vi "digital_demod_fpga.vi"() -> ()   [LabVIEW 2018]
uses:
  <vilib>/Platform/TimedLoop/XDataNode/timing_clust.ctl
  <vilib>/Platform/TimedLoop/XDataNode/nitl_modes.ctl
  <vilib>/Platform/TimedLoop/XDataNode/wakeup.ctl
  <vilib>/rvi/FXPMathLib/FxpAtan2/subVIs/nifxpmath_Atan2_SimConfig.ctl
  <vilib>/rvi/Emulation/niFpgaGetClockAttributes.vi
  <vilib>/rvi/Emulation/niFpgaSctlEmulationGetInTimedLoop.vi
  <vilib>/rvi/Emulation/niFpgaEmulationReportErrorSimple.vi
  <vilib>/rvi/Emulation/niFpgaCriticalErrorInLSC.vi
  <vilib>/rvi/Emulation/niFpgaProcessEmulError.vi
  <vilib>/rvi/eio/common/nirviEmuTemplateMethod_errors.vi
  <vilib>/rvi/DataTransferAndStorage/Container/Common/niFpgaContainerExecOnDevCompGetState.vi
  <vilib>/rvi/Emulation/niFpgaEmulationIsFPGAContextNoSignature.vi
  <vilib>/rvi/errors/niFpgaSetErrorForExecOnDevCompSimple.vi
  <vilib>/rvi/eio/common/nirviEmuReportErrorAndStop.vi
  <vilib>/rvi/DataTransferAndStorage/Container/Common/niFpgaContainerGetUniqueNameForEmu.vi
  <vilib>/rvi/FIFO/Fifo_Resource/nirvififoEmulationSetSize.vi
  <vilib>/rvi/FIFO/Fifo_Resource/nirviFifoEmulationQueueMgr.vi
  <instcachedir>/0/nirviFifoEmulationQueueMgr_E5CAEC123FF24DC58D834DCA3CDAA9B5.lvgen/nirviFifoEmulationQueueMgr_E5CAEC123FF24DC58D834DCA3CDAA9B5_006.vi
  <vilib>/rvi/FIFO/Fifo_Resource/nirvififoEmulationDetermineInputValidOut.vi
  <vilib>/rvi/FIFO/Fifo_Resource/nirvififoEmulationCreateLock.vi
  <vilib>/rvi/FIFO/Fifo_Resource/nirvififoEmulationObtainLock.vi
  <vilib>/rvi/FIFO/Fifo_Resource/nirvififoEmulationReleaseLock.vi
  <vilib>/rvi/occurrence/nirviWaitOnOccurrenceBase.vi
  <vilib>/rvi/errors/nirviReportUnexpectedCaseInternalError.vi
  <vilib>/rvi/errors/nirviReportUnexpectedCaseInternalError (U32).vi
  <vilib>/Utility/error.llb/Clear Errors.vi
  <vilib>/rvi/interface/RandomDataEmulation/niFpgaRandomDataHandleErrors.vi
  <instcachedir>/0/nirviFifoEmulationQueueMgr_E5CAEC123FF24DC58D834DCA3CDAA9B5.lvgen/nirviFifoEmulationQueueMgr_E5CAEC123FF24DC58D834DCA3CDAA9B5_001.vi
  <vilib>/rvi/Memory/Memory_Emulation/niFpgaMemoryEmulationCacheClearOnFirstRun.vi
  <vilib>/rvi/Memory/Memory_Emulation/nirvimemoryEmulationManagerCache_MakeExclusive.vi
  <vilib>/rvi/Memory/Memory_Emulation/niFpgaMemoryEmulationValidateCache.vi
  <vilib>/rvi/Memory/Memory_Emulation/nirvimemoryEmulationManagerCache_InsertValue.vi
  <vilib>/rvi/Memory/Memory_Emulation/nirvimemoryEmulationManagerCache_ReleaseExclusive.vi
  <vilib>/rvi/Memory/Memory_Emulation/nirvimemoryEmulationManagerCache_GetValue.vi
  <vilib>/rvi/Memory/Memory_Emulation/nirvimemoryEmulationManagerCache_SetValue.vi
  <vilib>/rvi/Emulation/niFpgaSctlEmulationResourceMgr.vi
  <instcachedir>/0/nirviFifoEmulationQueueMgr_E5CAEC123FF24DC58D834DCA3CDAA9B5.lvgen/nirviFifoEmulationQueueMgr_E5CAEC123FF24DC58D834DCA3CDAA9B5_003.vi
  <instcachedir>/0/nirviFifoEmulationQueueMgr_E5CAEC123FF24DC58D834DCA3CDAA9B5.lvgen/nirviFifoEmulationQueueMgr_E5CAEC123FF24DC58D834DCA3CDAA9B5_002.vi
  <instcachedir>/0/nirviFifoEmulationQueueMgr_E5CAEC123FF24DC58D834DCA3CDAA9B5.lvgen/nirviFifoEmulationQueueMgr_E5CAEC123FF24DC58D834DCA3CDAA9B5_004.vi
  <vilib>/rvi/FXPMathLib/FxpAtan2/simVIs/DllFxpAtan2Temp_sub.vi
  <instcachedir>/0/nirviFifoEmulationQueueMgr_E5CAEC123FF24DC58D834DCA3CDAA9B5.lvgen/nirviFifoEmulationQueueMgr_E5CAEC123FF24DC58D834DCA3CDAA9B5_009.vi
  <instcachedir>/0/nirviFifoEmulationQueueMgr_E5CAEC123FF24DC58D834DCA3CDAA9B5.lvgen/nirviFifoEmulationQueueMgr_E5CAEC123FF24DC58D834DCA3CDAA9B5_007.vi
  <instcachedir>/0/nirviFifoEmulationQueueMgr_E5CAEC123FF24DC58D834DCA3CDAA9B5.lvgen/nirviFifoEmulationQueueMgr_E5CAEC123FF24DC58D834DCA3CDAA9B5_008.vi
  <vilib>/Platform/TimedLoop/XDataNode/XDataNode.xnode
  <vilib>/eio/EIONode/EIONode.xnode
  <vilib>/rvi/DataTransferAndStorage/Container/XNode/niFpgaContainer.xnode
  <vilib>/rvi/FIFO/Fifo_Resource/niFpgaFifoEmulationRefIn.vi
  <vilib>/rvi/Memory/Memory_Emulation/niFpgaMemoryEmulationRefIn.vi
  <vilib>/rvi/FXPMathLib/FxpInterpret/XNode/nifxpmath_Interpret.xnode
  <vilib>/rvi/FXPMathLib/FxpAtan2/XNode/nifxpmath_Atan2.xnode
  <vilib>/Platform/TimedLoop/XDataNode/XDNodeRunTimeDep.lvlib
  FPGA Timekeeper 1.1b0/FPGA Timekeeper.lvlib
  <instrlib>/_niInstr_jank/Basic Elements/v1/FPGA/niInstr Basic Elements v1 FPGA.lvlib
panel:
  in  "sum_z-pow_fb":bool
  in  "pow_dc_offset":i16
  out "pow_set_actual":fxp<+/-,33,33>
  in  "fb_on_pow_set":bool
  in  "pow_fb":bool
  in  "pow_lower_lim":i16
  in  "pow_upper_lim":i16
  in  "pow_pg":fxp<+/-,32,16>
  in  "pow_dg":fxp<+/-,32,16>
  out "amp4_lf":i32
  out "delta_pow_set":fxp<+/-,32,32>
  in  "delta_pow_set_llim":fxp<+/-,32,32>
  in  "delta_pow_set_ulim":fxp<+/-,32,32>
  out "pow_shifted":i32
  in  "pow_fb_bitshift":i16
  in  "reset_pow_accum":bool
  in  "pow_ig":fxp<+/-,32,16>
  in  "pow_set_user":fxp<+/-,32,32>
  in  "pow_bitshift":i16
  out "z_fb_tot_i16":i16
  in  "z_internal_inject_scale":i16
  in  "add_sin":bool
  in  "z_internal_inject_freq":fxp<+,32,0>=0.0002500000409781933
  in  "inject_sigs":bool
  in  "downsample->xyz":bool=TRUE
  in  "xy2_bitshift":i16
  in  "TRIG0":bool
  in  "block_config_trig":bool
  out "DIO22":bool
  in  "trig_loop_timer (usec)":u32=2
  out "config_trig":bool
  in  "reset_config_trig":bool
  in  "manual_config_trig":bool
  out "x_fb_i16":i16
  in  "z_lower_lim":i16
  in  "z_upper_lim":i16
  in  "y_lower_lim":i16
  in  "y_upper_lim":i16
  in  "x_lower_lim":i16
  in  "x_upper_lim":i16
  in  "reset_z_accum":bool
  in  "z_ig":fxp<+/-,32,16>
  in  "z_pg":fxp<+/-,32,16>
  in  "z_fb_bitshift":i16
  in  "z_dg":fxp<+/-,32,16>
  in  "z_set_user":fxp<+/-,32,32>
  out "z_shifted":i32
  in  "y_dg":fxp<+/-,32,16>
  in  "xy_fb_bitshift":i16
  in  "x_dg":fxp<+/-,32,16>
  out "y_shifted":i32
  in  "z_bitshift":i16
  out "x_shifted":i32
  in  "xy_bitshift":i16
  out "z_fb_i16":i16
  out "y_fb_i16":i16
  in  "z_dc_offset":i16
  in  "y_dc_offset":i16
  in  "x_dc_offset":i16
  in  "RT time (ns)":u64
  out "time (ns)":u64
  in  "reset_phi4":bool
  in  "reset_phi3":bool
  in  "reset_phi2":bool
  in  "reset_phi1":bool
  out "phi4_full_out":fxp<+/-,32,18> format="%.15g"
  out "n4":i16
  out "amp4_out":fxp<+,32,16> format="%.23g"
  out "sig4":i16
  in  "downsamp_num":i16=100
  out "phi3_full_out":fxp<+/-,32,18> format="%.15g"
  out "n3":i16
  out "phi2_full_out":fxp<+/-,32,18> format="%.15g"
  out "n2":i16
  out "phi1_full_out":fxp<+/-,32,18> format="%.15g"
  out "n1":i16
  out "sig3":i16
  out "sig2":i16
  out "sig1":i16
  out "amp0_out":fxp<+,32,16>
  out "amp1_out":fxp<+,32,16>
  out "amp2_out":fxp<+,32,16>
  in  "subtract_mean":bool
  out "sig0":i16
  in  "discont_pos":fxp<+/-,17,3>=1.0
  in  "discont_neg":fxp<+/-,3,2>=-1.0
  in  "reset_phi0":bool
  out "amp3_out":fxp<+,32,16> format="%.23g"
  out "phi0_full_out":fxp<+/-,32,18> format="%.15g"
  out "n0":i16
  out "loop time":fxp<+,32,32> format="%.39g"
  in  "loop timer (usec)":u32=2
  in  "Counter Offset":u8
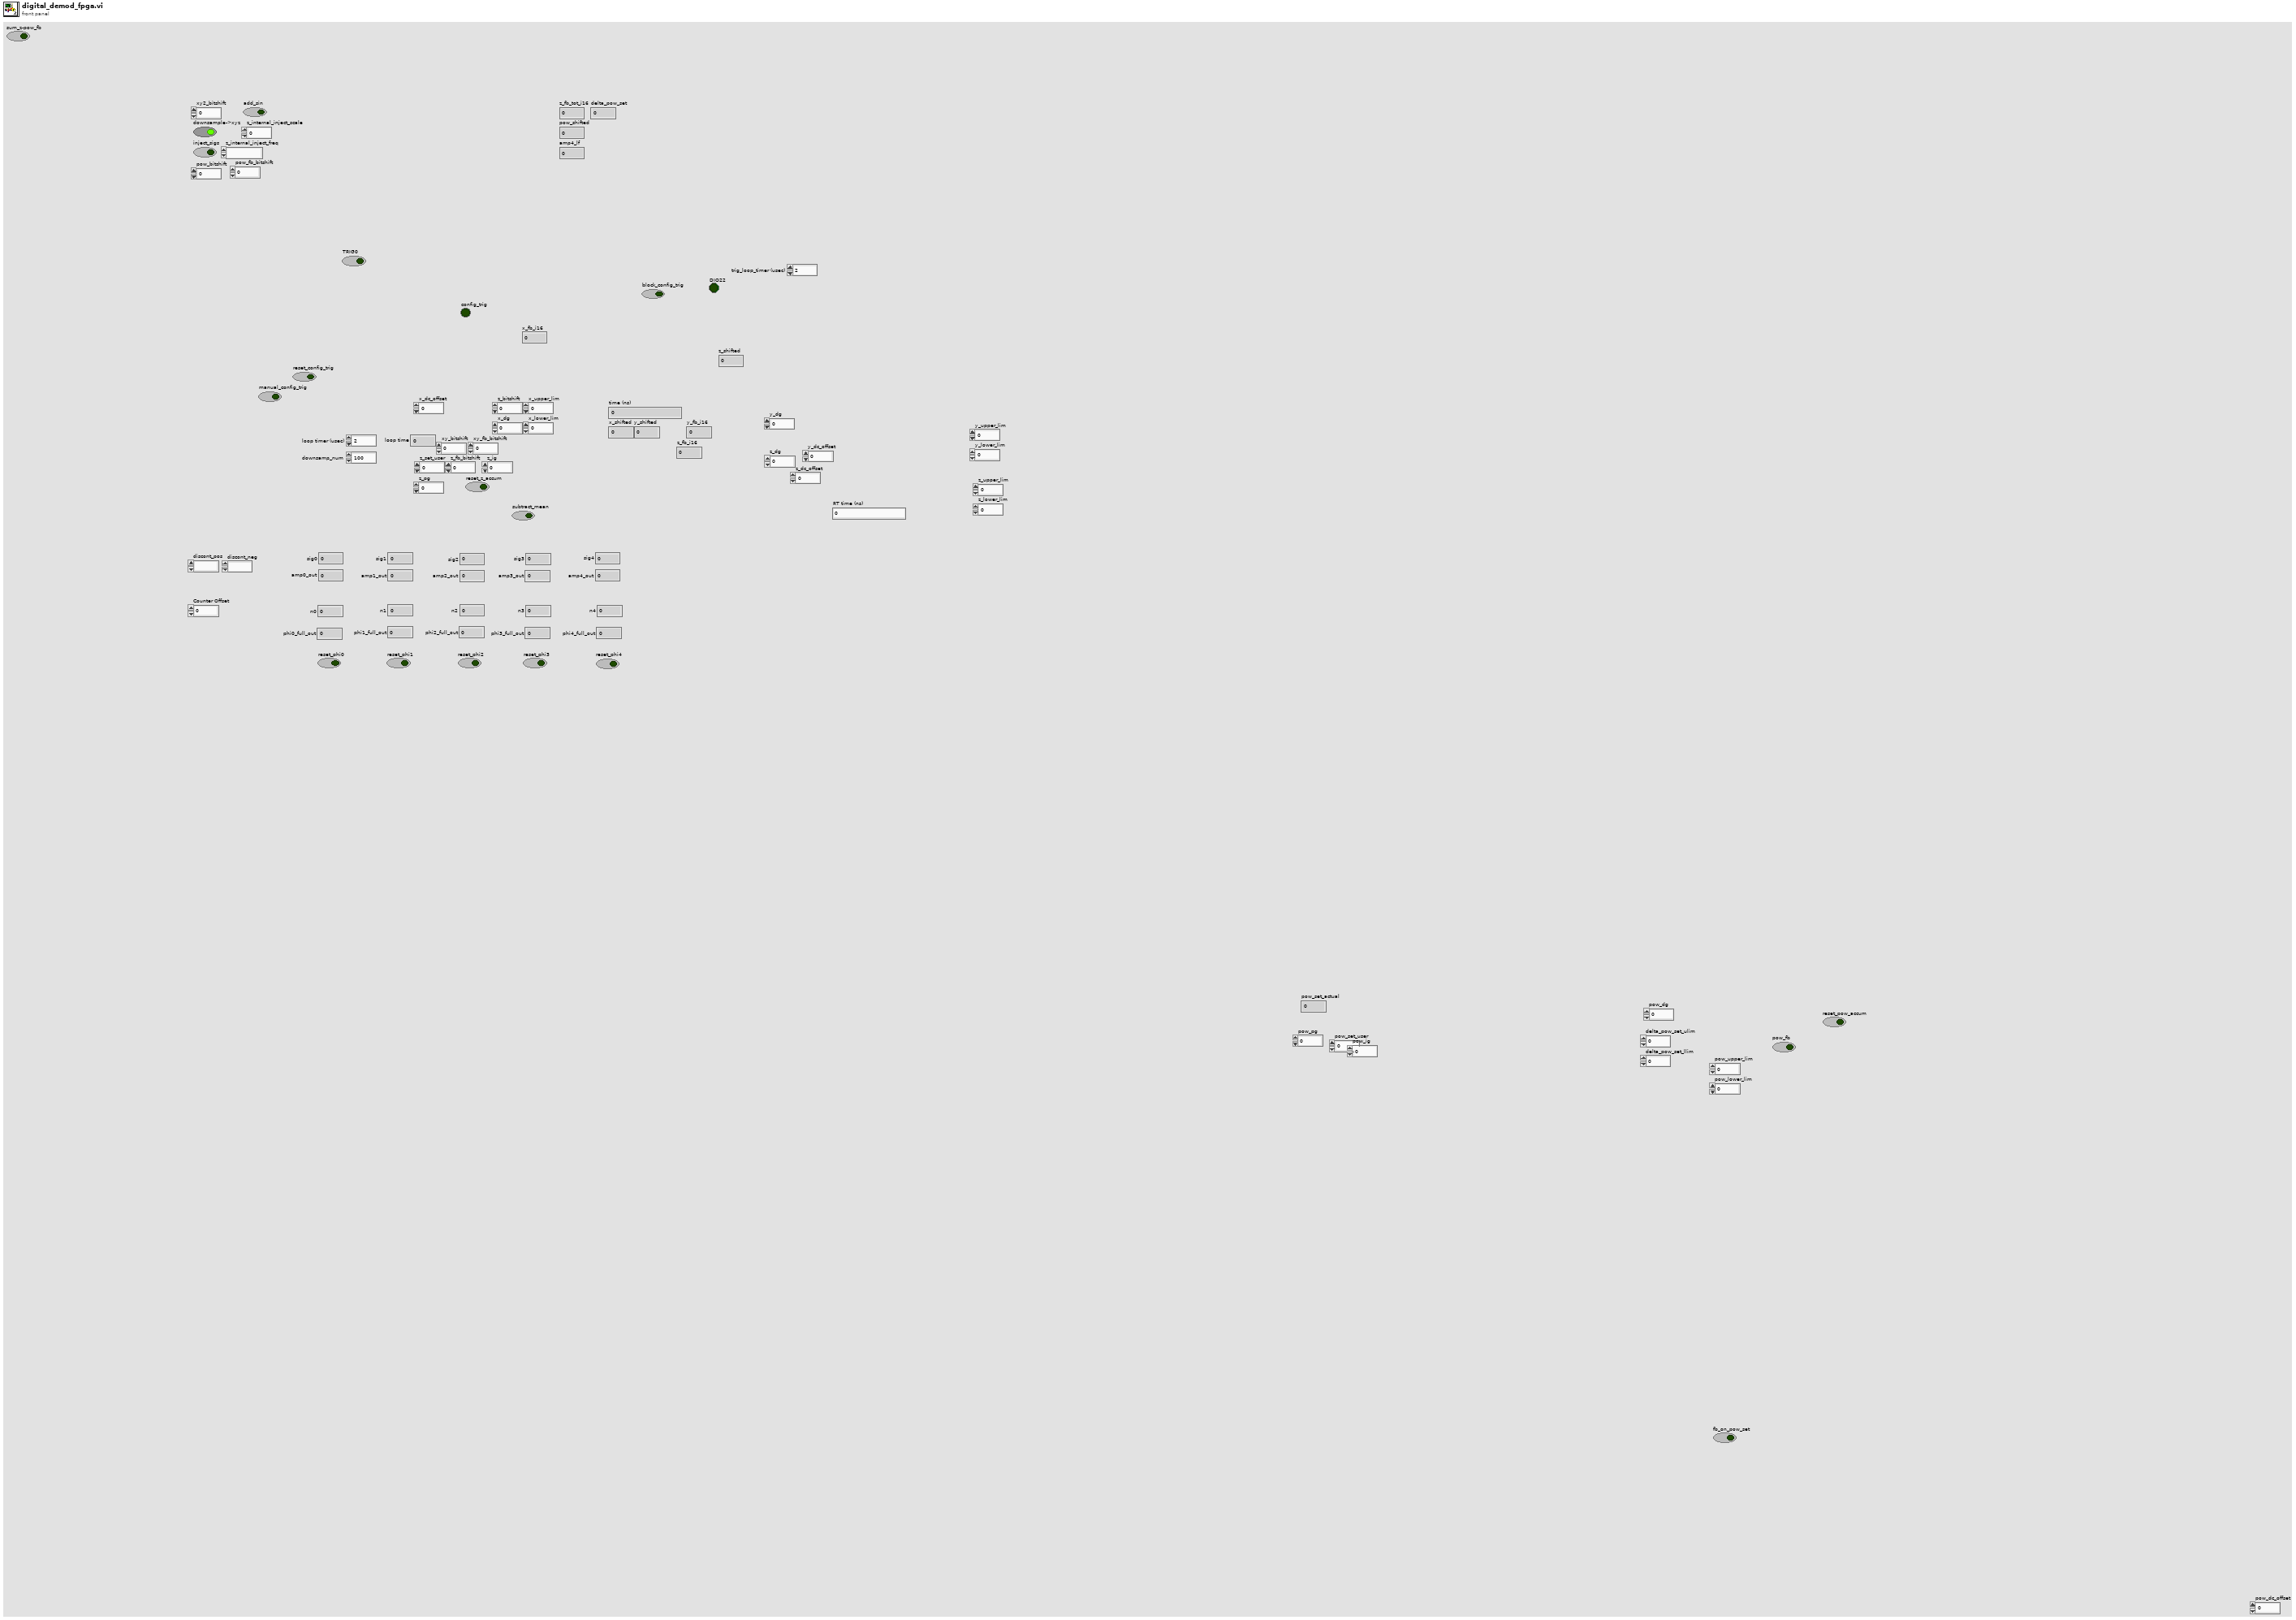
[diagram p1: front panel]
types:
  T1 = typedef "XDNodeRunTimeDep.lvlib/timing_clust.ctl" = cluster{"Expected End [f-1]":u64, "Actual End [f-1]":u64, "Finished Late? [f-1]":bool, "Expected End [i-1]":u64, "Actual End [i-1]":u64, "Finished Late? [i-1]":bool, "Expected Start [i]":u64, "Actual Start [i]":u64, "Expected Start [f]":u64, "Actual Start [f]":u64, "Source Name":string, "Structure Name":string, "Period":i64, "Deadline":i64, "Offset":i64, "Start":i64, "Priority":i32, "Timeout":i32, "Mode":T2, "Wakeup Reason":T3, "Error":errorcluster, "Source Type":string, "Secondary Source Type":string, "Global End Time":u64, "Global Start Time":u64, "Frame Duration":u64, "Iteration Duration":u64, "Assigned CPU":i32, "I/O Scan Engine Mode":u32}
  T2 = typedef "XDNodeRunTimeDep.lvlib/nitl_modes.ctl" = enum32{"No Change", "Process missed periods, maintain original phase", "Discard missed periods, maintain original phase", "Process missed periods, ignore original phase", "Discard missed periods, ignore original phase"}
  T3 = typedef "XDNodeRunTimeDep.lvlib/wakeup.ctl" = enum32{"Normal", "Aborted", "Asynchronous wakeup", "Timing source error", "Timed loop error", "Timeout"}
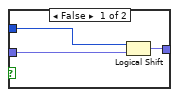
[diagram p5: hidden frame]
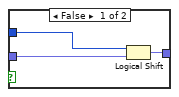
[diagram p6: hidden frame]
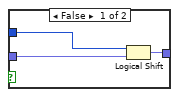
[diagram p7: hidden frame]
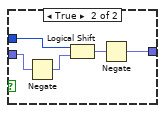
[diagram p9: hidden frame]
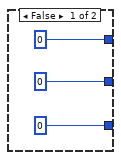
[diagram p11: hidden frame]
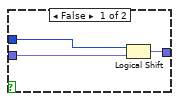
[diagram p13: hidden frame]
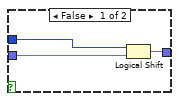
[diagram p14: hidden frame]
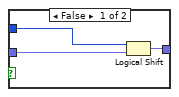
[diagram p15: hidden frame]
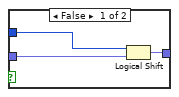
[diagram p16: hidden frame]
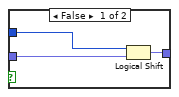
[diagram p17: hidden frame]
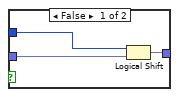
[diagram p18: hidden frame]
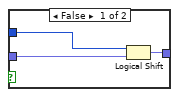
[diagram p19: hidden frame]
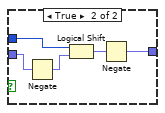
[diagram p20: hidden frame]
diagram:
  n1 = flat-sequence {
    frame #0 {
    }
    frame #1 {
      w5 = i16 0
      w18 = refnum<k21> "20MHz"  # FPGA Clock
      n2 = call "Timekeeper.vi"() -> ()  [unwired: 12 in]
      n3 = while {
        shift-right: [w684] -> _
        shift-left: u8 0 -> [w682]
        shift-right: [w677] -> _
        shift-left: u16 0 -> [w681]
        shift-right: [w676] -> _
        shift-left: 0 -> [w678]
        shift-right: [w673] -> _
        shift-left: 0 -> [w674]
        shift-right: [w670] -> _
        shift-left: 0 -> [w671]
        shift-right: [w667] -> _
        shift-left: 0 -> [w668]
        shift-right: [w666] -> _
        shift-left: _ -> [w664]
        shift-right: [w662] -> _
        shift-left: _ -> [w658]
        shift-right: [w663] -> _
        shift-left: _ -> [w660]
        shift-right: [w656] -> _
        shift-left: _ -> [w654]
        shift-right: [w657] -> _
        shift-left: _ -> [w643]
        shift-right: [w652] -> _
        shift-left: w5 -> [w650]
        shift-right: [w646] -> _
        shift-left: _ -> [w629]
        shift-right: [w640] -> _
        shift-left: 0 -> [w641]
        shift-right: [w631] -> _
        shift-left: w5 -> [w638]
        shift-right: [w632] -> _
        shift-left: w5 -> [w637]
        shift-right: [w633] -> _
        shift-left: w5 -> [w636]
        shift-right: [w634] -> _
        shift-left: w5 -> [w635]
        stop <- FALSE ("Stop") stop-if-true
        n4 = flat-sequence {
          tunnel: [w706] -> w683
          tunnel: w682 -> [w706]
          tunnel: w681 -> [w705]
          tunnel: [w704] -> w680
          tunnel: [w703] -> w679
          tunnel: w678 -> [w703]
          tunnel: [w702] -> w675
          tunnel: w674 -> [w702]
          tunnel: [w701] -> w672
          tunnel: w671 -> [w701]
          tunnel: [w700] -> w669
          tunnel: w668 -> [w700]
          tunnel: [w699] -> w665
          tunnel: w664 -> [w699]
          tunnel: [w698] -> w661
          tunnel: w660 -> [w698]
          tunnel: [w697] -> w659
          tunnel: w658 -> [w697]
          tunnel: [w696] -> w655
          tunnel: w643 -> [w696]
          tunnel: w654 -> [w695]
          tunnel: [w695] -> w653
          tunnel: [w694] -> w651
          tunnel: w650 -> [w694]
          tunnel: [w693] -> w649
          tunnel: w638 -> [w693]
          tunnel: [w692] -> w648
          tunnel: w637 -> [w692]
          tunnel: [w688] -> w647
          tunnel: w636 -> [w688]
          tunnel: [w691] -> w645
          tunnel: w629 -> [w691]
          tunnel: [w690] -> w644
          tunnel: w643 -> [w690]
          tunnel: [w689] -> w642
          tunnel: w641 -> [w689]
          tunnel: [w687] -> w639
          tunnel: w635 -> [w687]
          tunnel: [w686] -> w630
          tunnel: w629 -> [w686]
          tunnel: [w968] -> w684
          tunnel: w683 -> [w967]
          tunnel: w680 -> [w723]
          tunnel: w679 -> [w715]
          tunnel: [w722] -> w677
          tunnel: [w947] -> w676
          tunnel: w675 -> [w721]
          tunnel: [w916] -> w673
          tunnel: w672 -> [w719]
          tunnel: [w915] -> w670
          tunnel: w669 -> [w717]
          tunnel: [w914] -> w667
          tunnel: [w909] -> w666
          tunnel: w665 -> [w908]
          tunnel: [w894] -> w663
          tunnel: [w893] -> w662
          tunnel: w661 -> [w892]
          tunnel: w659 -> [w891]
          tunnel: [w853] -> w657
          tunnel: [w852] -> w656
          tunnel: w655 -> [w708]
          tunnel: w653 -> [w851]
          tunnel: [w850] -> w652
          tunnel: w651 -> [w836]
          tunnel: w649 -> [w835]
          tunnel: w648 -> [w810]
          tunnel: w647 -> [w809]
          tunnel: [w804] -> w646
          tunnel: w645 -> [w707]
          tunnel: w644 -> [w803]
          tunnel: w642 -> [w713]
          tunnel: [w791] -> w640
          tunnel: w639 -> [w760]
          tunnel: [w755] -> w634
          tunnel: [w754] -> w633
          tunnel: [w753] -> w632
          tunnel: [w752] -> w631
          tunnel: w630 -> [w749]
          frame #0 {
            n5 = Increment(x=w705) -> (x+1=w704:u16)
          }
          frame #1 {
            w735 = refnum<k21> "x_hf"  # FIFO
            w736 = refnum<k21> "y_hf"  # FIFO
            w751 = refnum<k21> "z_hf"  # FIFO
            w798 = refnum<k21> "chan4_moving_avg"  # Memory
            w750 = 0
            w925 = refnum<k21> "chan2_moving_avg"  # Memory
            w931 = refnum<k21> "chan1_moving_avg"  # Memory
            w937 = refnum<k21> "chan0_moving_avg"  # Memory
            w950 = refnum<k21> "chan3_moving_avg"  # Memory
            # "Multiply n by 2 (since phase is in pi*radians)\nand cast to FXP via FXP reinterpretation"
            # "Divide by 4096 = 2^12 \nvia FXP reinterpretation"
            # "Divide by 4096 = 2^12 \nvia FXP reinterpretation"
            # "Divide by 4096 = 2^12 \nvia FXP reinterpretation"
            # "Divide by 4096 = 2^12 \nvia FXP reinterpretation"
            # "Divide by 4096 = 2^12 \nvia FXP reinterpretation"
            # "Cast to (+12,12) with overflow\noption set to wrap (outputs \n0 -> 4095) then back to U16"
            # "delay amplitude by one adc cycle to match with phase"
            n6 = Index Array(array=w803) -> (element #1=w799:fxp<+,32,16>, element #2=w801:fxp<+,32,16>, element #3=w800:fxp<+,32,16>, element #4=w802:fxp<+,32,16>)  [unwired: 4 in]
            n7 = To Fixed-Point(number=w723) -> (fixed-point=w724:fxp<+,12,12>)  [unwired: 1 in]
            n8 = for {
              N: 5 -> [_]
              tunnel: [w1150] -> w907 mode=indexing
              w1152 = refnum<k21> "acq_data"  # FIFO
              n9 = xnode ("FIFO Read")("Timeout"=i16 -1, "FIFO In"=w1152) -> ("Element"=w1150:i16)  [unwired: 2 out]
            }
            n10 = Index Array(array=w749, index=i16 4) -> (element=w747:fxp<+/-,32,18>)
            n11 = Add(x="Counter Offset", y=w967) -> (x+y=w711:u8)
            n12 = To Unsigned Word Integer(number=w724) -> (unsigned 16bit integer=w722:u16)
            n13 = Index Array(array=w851) -> (element #1=w837:fxp<+/-,16,2>, element #2=w838:fxp<+/-,16,2>, element #3=w812:fxp<+/-,16,2>, element #4=w811:fxp<+/-,16,2>, element #5=w762:fxp<+/-,16,2>)  [unwired: 5 in]
            n14 = Index Array(array=w892) -> (element #1=w875:i16, element #2=w873:i16, element #3=w871:i16, element #4=w869:i16, element #5=w778:i16)  [unwired: 5 in]
            n15 = Index Array(array=w891) -> (element #1=w874:i16, element #2=w872:i16, element #3=w870:i16, element #4=w868:i16, element #5=w779:i16)  [unwired: 5 in]
            n16 = Add(x=w799, y=w801) -> (x+y=w743:fxp<+,33,17>)
            n17 = Add(x=w800, y=w802) -> (x+y=w744:fxp<+,33,17>)
            n18 = Add(x=w799, y=w800) -> (x+y=w746:fxp<+,33,17>)
            n19 = Add(x=w801, y=w802) -> (x+y=w745:fxp<+,33,17>)
            n20 = Quotient & Remainder(x=w711, y=u8 4) -> (x-y*floor(x/y)=w709:u8)  [unwired: 1 out]
            n21 = Subtract(x=w743, y=w744) -> (x-y=w740:fxp<+/-,34,18>)
            n22 = Add(x=w743, y=w744) -> (x+y=w739:fxp<+,34,18>)
            n23 = Subtract(x=w746, y=w745) -> (x-y=w742:fxp<+/-,34,18>)
            n24 = Add(x=w746, y=w745) -> (x+y=w741:fxp<+,34,18>)
            n25 = Divide(x=w742, y=w741) -> (x/y=w737:fxp<+/-,64,32>)
            n26 = Divide(x=w740, y=w739) -> (x/y=w738:fxp<+/-,64,32>)
            n27 = To Fixed-Point(number=w875) -> (fixed-point=w877:fxp<+/-,16,16>)  [unwired: 1 in]
            n28 = To Fixed-Point(number=w874) -> (fixed-point=w876:fxp<+/-,16,16>)  [unwired: 1 in]
            n29 = Index Array(array=w907) -> (element #1=w917:i16, element #2=w918:i16, element #3=w919:i16, element #4=w895:i16, element #5=w792:i16)  [unwired: 5 in]
            n30 = for {
              tunnel: w708 -> [w974] mode=indexing
              w976 = refnum<k21> "amp_hf"  # FIFO
              n31 = xnode ("FIFO Write")("Element"=w974, "Timeout"=0, "FIFO In"=w976) -> ()  [unwired: 2 out]
            }
            n32 = xnode "High Throughput Inverse Tangent (2 Input)"("y"=w877, "x"=w876) -> ("atan2(y,x) (pi)"=w867:fxp<+/-,16,2>)
            n33 = To Fixed-Point(number=w873) -> (fixed-point=w882:fxp<+/-,16,16>)  [unwired: 1 in]
            n34 = To Fixed-Point(number=w872) -> (fixed-point=w881:fxp<+/-,16,16>)  [unwired: 1 in]
            n35 = feedback #1() -> (w936:u16)  [unwired: 1 in]
            n36 = feedback-in #1(w722) -> ()
            n37 = feedback #2() -> (w941:fxp<+/-,16,2>)  [unwired: 1 in]
            n38 = feedback-in #2(w837) -> ()
            n39 = feedback #3() -> (w839:fxp<+/-,16,2>)  [unwired: 1 in]
            n40 = feedback-in #3(w838) -> ()
            n41 = feedback #4() -> (w824:fxp<+/-,16,2>)  [unwired: 1 in]
            n42 = feedback-in #4(w812) -> ()
            n43 = xnode "Reinterpret Number"("x"=w721) -> ("y"=w720:fxp<+/-,32,20>)
            n44 = feedback #5() -> (w813:fxp<+/-,16,2>)  [unwired: 1 in]
            n45 = feedback-in #5(w811) -> ()
            n46 = feedback #6() -> (w765:fxp<+/-,16,2>)  [unwired: 1 in]
            n47 = feedback-in #6(w762) -> ()
            n48 = Subtract(x=w941, y=w837) -> (x-y=w951:fxp<+/-,17,3>)
            n49 = Subtract(x=w839, y=w838) -> (x-y=w840:fxp<+/-,17,3>)
            n50 = Subtract(x=w824, y=w812) -> (x-y=w825:fxp<+/-,17,3>)
            n51 = Subtract(x=w813, y=w811) -> (x-y=w814:fxp<+/-,17,3>)
            n52 = Subtract(x=w765, y=w762) -> (x-y=w766:fxp<+/-,17,3>)
            n53 = xnode "High Throughput Inverse Tangent (2 Input)"("y"=w882, "x"=w881) -> ("atan2(y,x) (pi)"=w866:fxp<+/-,16,2>)
            n54 = To Fixed-Point(number=w871) -> (fixed-point=w887:fxp<+/-,16,16>)  [unwired: 1 in]
            n55 = To Fixed-Point(number=w870) -> (fixed-point=w886:fxp<+/-,16,16>)  [unwired: 1 in]
            n56 = case shown="True" "subtract_mean" {
              tunnel: [w1101 w1119] -> w946
              tunnel: w908 -> [_ w1117]
              tunnel: w907 -> [w1102 w1118]
              tunnel: [w1100 w1108] -> w854
              tunnel: [w1099 w1107] -> w855
              tunnel: [w1098 w1106] -> w856
              tunnel: [w1097 w1103] -> w789
              frame False {
                n57 = Index Array(array=w1102) -> (element #1=w1101:i16, element #2=w1100:i16, element #3=w1099:i16, element #4=w1098:i16, element #5=w1097:i16)  [unwired: 5 in]
              }
              frame True {
                n58 = Index Array(array=w1117) -> (element #1=w1109:i16, element #2=w1110:i16, element #3=w1111:i16, element #4=w1112:i16, element #5=w1104:i16)  [unwired: 5 in]
                n59 = Index Array(array=w1118) -> (element #1=w1116:i16, element #2=w1115:i16, element #3=w1114:i16, element #4=w1113:i16, element #5=w1105:i16)  [unwired: 5 in]
                n60 = Subtract(x=w1116, y=w1109) -> (x-y=w1119:i16)
                n61 = Subtract(x=w1115, y=w1110) -> (x-y=w1108:i16)
                n62 = Subtract(x=w1114, y=w1111) -> (x-y=w1107:i16)
                n63 = Subtract(x=w1113, y=w1112) -> (x-y=w1106:i16)
                n64 = Subtract(x=w1105, y=w1104) -> (x-y=w1103:i16)
              }
            }
            "sig0" <- w946
            "sig1" <- w854
            "sig2" <- w855
            "sig3" <- w856
            "sig4" <- w789
            n65 = Square(x=w877) -> (x^2=w878:fxp<+,31,31>)
            n66 = Square(x=w876) -> (x^2=w879:fxp<+,31,31>)
            n67 = xnode ("Memory Write")("Address"=w936, "Data"=w917, "Memory In"=w937) -> ()  [unwired: 1 out]
            n68 = Add(x=w878, y=w879) -> (x+y=w880:fxp<+,32,32>)
            n69 = To Long Integer(number=w917) -> (32bit integer=w934:i32)
            n70 = for {
              tunnel: w707 -> [w972] mode=indexing
              w973 = refnum<k21> "phi_hf"  # FIFO
              n71 = xnode ("FIFO Write")("Element"=w972, "Timeout"=0, "FIFO In"=w973) -> ()  [unwired: 2 out]
            }
            n72 = xnode ("FIFO Write")("Element"=w738, "Timeout"=w750, "FIFO In"=w735) -> ()  [unwired: 2 out]
            n73 = feedback #7() -> (w930:u16)  [unwired: 1 in]
            n74 = feedback-in #7(w722) -> ()
            n75 = Square Root(x=w880) -> (sqrt(x)=w863:fxp<+,32,16>)
            n76 = xnode "Reinterpret Number"("x"=w719) -> ("y"=w718:fxp<+/-,32,20>)
            n77 = xnode "High Throughput Inverse Tangent (2 Input)"("y"=w887, "x"=w886) -> ("atan2(y,x) (pi)"=w865:fxp<+/-,16,2>)
            n78 = Add(x=w721, y=w934) -> (x+y=w935:i32)
            n79 = To Fixed-Point(number=w869) -> (fixed-point=w940:fxp<+/-,16,16>)  [unwired: 1 in]
            n80 = To Fixed-Point(number=w868) -> (fixed-point=w939:fxp<+/-,16,16>)  [unwired: 1 in]
            n81 = Square(x=w882) -> (x^2=w883:fxp<+,31,31>)
            n82 = Square(x=w881) -> (x^2=w884:fxp<+,31,31>)
            n83 = Less?(x=w951, y="discont_neg") -> (x < y?=w953:bool)
            n84 = Greater?(x=w951, y="discont_pos") -> (0:w957:bool)
            n85 = Less?(x=w840, y="discont_neg") -> (x < y?=w842:bool)
            n86 = Greater?(x=w840, y="discont_pos") -> (0:w846:bool)
            n87 = Less?(x=w825, y="discont_neg") -> (x < y?=w827:bool)
            n88 = Greater?(x=w825, y="discont_pos") -> (0:w831:bool)
            n89 = Less?(x=w814, y="discont_neg") -> (x < y?=w816:bool)
            n90 = Greater?(x=w814, y="discont_pos") -> (0:w820:bool)
            n91 = Less?(x=w766, y="discont_neg") -> (x < y?=w768:bool)
            n92 = Greater?(x=w766, y="discont_pos") -> (0:w772:bool)
            n93 = feedback #8() -> (w860:fxp<+,32,16>)  [unwired: 1 in]
            "amp0_out" <- w860
            n94 = feedback-in #8(w863) -> ()
            n95 = Add(x=w883, y=w884) -> (x+y=w885:fxp<+,32,32>)
            n96 = xnode ("Memory Write")("Address"=w930, "Data"=w918, "Memory In"=w931) -> ()  [unwired: 1 out]
            n97 = xnode "High Throughput Inverse Tangent (2 Input)"("y"=w940, "x"=w939) -> ("atan2(y,x) (pi)"=w864:fxp<+/-,16,2>)
            n98 = Square Root(x=w885) -> (sqrt(x)=w862:fxp<+,32,16>)
            n99 = Select(t=i16 -1, s=w953, f=i16 0) -> (s? t:f=w958:i16)
            n100 = Select(t=i16 -1, s=w842, f=i16 0) -> (s? t:f=w847:i16)
            n101 = Select(t=i16 -1, s=w827, f=i16 0) -> (s? t:f=w832:i16)
            n102 = Select(t=i16 -1, s=w816, f=i16 0) -> (s? t:f=w821:i16)
            n103 = Select(t=i16 -1, s=w768, f=i16 0) -> (s? t:f=w773:i16)
            n104 = xnode ("Memory Read")("Address"=w722, "Memory In"=w937) -> ("Data"=w932:i16)  [unwired: 1 out]
            n105 = To Long Integer(number=w918) -> (32bit integer=w928:i32)
            n106 = To Word Integer(number=w720) -> (16bit integer=w910:i16)
            n107 = To Fixed-Point(number=w778) -> (fixed-point=w782:fxp<+/-,16,16>)  [unwired: 1 in]
            n108 = To Fixed-Point(number=w779) -> (fixed-point=w781:fxp<+/-,16,16>)  [unwired: 1 in]
            n109 = Square(x=w887) -> (x^2=w888:fxp<+,31,31>)
            n110 = Square(x=w886) -> (x^2=w889:fxp<+,31,31>)
            n111 = feedback #9() -> (w924:u16)  [unwired: 1 in]
            n112 = feedback-in #9(w722) -> ()
            n113 = Select(t=i16 1, s=w957, f=i16 0) -> (s? t:f=w959:i16)
            n114 = Select(t=i16 1, s=w846, f=i16 0) -> (s? t:f=w848:i16)
            n115 = Select(t=i16 1, s=w831, f=i16 0) -> (s? t:f=w833:i16)
            n116 = Select(t=i16 1, s=w820, f=i16 0) -> (s? t:f=w822:i16)
            n117 = Select(t=i16 1, s=w772, f=i16 0) -> (s? t:f=w774:i16)
            n118 = Add(x=w719, y=w928) -> (x+y=w929:i32)
            n119 = Add(x=w888, y=w889) -> (x+y=w890:fxp<+,32,32>)
            n120 = xnode "Reinterpret Number"("x"=w717) -> ("y"=w716:fxp<+/-,32,20>)
            n121 = feedback #10() -> (w859:fxp<+,32,16>)  [unwired: 1 in]
            "amp1_out" <- w859
            n122 = feedback-in #10(w862) -> ()
            n123 = Add(x=w958, y=w959) -> (x+y=w960:i16)
            n124 = Add(x=w847, y=w848) -> (x+y=w849:i16)
            n125 = Add(x=w832, y=w833) -> (x+y=w834:i16)
            n126 = xnode ("FIFO Write")("Element"=w737, "Timeout"=w750, "FIFO In"=w736) -> ()  [unwired: 2 out]
            n127 = Add(x=w821, y=w822) -> (x+y=w823:i16)
            n128 = Add(x=w773, y=w774) -> (x+y=w775:i16)
            n129 = Square Root(x=w890) -> (sqrt(x)=w861:fxp<+,32,16>)
            n130 = feedback #11() -> (w949:u16)  [unwired: 1 in]
            n131 = feedback-in #11(w722) -> ()
            n132 = xnode "High Throughput Inverse Tangent (2 Input)"("y"=w782, "x"=w781) -> ("atan2(y,x) (pi)"=w777:fxp<+/-,16,2>)
            n133 = xnode "Reinterpret Number"("x"=w715) -> ("y"=w714:fxp<+/-,32,20>)
            n134 = Add(x=w836, y=w960) -> (x+y=w734:i16)
            "n0" <- w734
            n135 = Square(x=w940) -> (x^2=w963:fxp<+,31,31>)
            n136 = Square(x=w939) -> (x^2=w964:fxp<+,31,31>)
            n137 = Add(x=w835, y=w849) -> (x+y=w732:i16)
            "n1" <- w732
            n138 = Add(x=w810, y=w834) -> (x+y=w726:i16)
            "n2" <- w726
            n139 = Add(x=w809, y=w823) -> (x+y=w727:i16)
            "n3" <- w727
            n140 = Add(x=w760, y=w775) -> (x+y=w730:i16)
            "n4" <- w730
            n141 = feedback #12() -> (w970:i16)  [unwired: 1 in]
            n142 = feedback-in #12(w946) -> ()
            n143 = xnode ("Memory Write")("Address"=w924, "Data"=w919, "Memory In"=w925) -> ()  [unwired: 1 out]
            n144 = feedback #13() -> (w906:i16)  [unwired: 1 in]
            n145 = feedback-in #13(w854) -> ()
            n146 = feedback #14() -> (w858:fxp<+,32,16>)  [unwired: 1 in]
            "amp2_out" <- w858
            n147 = feedback-in #14(w861) -> ()
            n148 = feedback #15() -> (w905:i16)  [unwired: 1 in]
            n149 = feedback-in #15(w855) -> ()
            n150 = feedback #16() -> (w904:i16)  [unwired: 1 in]
            n151 = feedback-in #16(w856) -> ()
            n152 = feedback #17() -> (w788:i16)  [unwired: 1 in]
            n153 = feedback-in #17(w789) -> ()
            n154 = xnode ("Memory Read")("Address"=w722, "Memory In"=w931) -> ("Data"=w926:i16)  [unwired: 1 out]
            n155 = To Long Integer(number=w919) -> (32bit integer=w922:i32)
            n156 = Add(x=w963, y=w964) -> (x+y=w965:fxp<+,32,32>)
            n157 = To Word Integer(number=w718) -> (16bit integer=w911:i16)
            n158 = feedback #18() -> (w797:u16)  [unwired: 1 in]
            n159 = feedback-in #18(w722) -> ()
            n160 = xnode "Reinterpret Number"("x"=w713) -> ("y"=w712:fxp<+/-,32,20>)
            n161 = Square Root(x=w965) -> (sqrt(x)=w938:fxp<+,32,16>)
            n162 = case shown="3" w709 {
              tunnel: w946 -> [w1162 w1177 w1194 w1212]
              tunnel: w970 -> [w1157 w1175 w1197 w1207]
              tunnel: [w1157 w1176 w1196 w1212] -> w902
              tunnel: [w1162 w1175 w1193 w1206] -> w903
              tunnel: w856 -> [w1159 w1168 w1185 w1209]
              tunnel: w855 -> [w1160 w1171 w1189 w1210]
              tunnel: w854 -> [w1161 w1174 w1195 w1211]
              tunnel: w906 -> [w1156 w1172 w1191 w1205]
              tunnel: w905 -> [w1155 w1169 w1187 w1203]
              tunnel: w904 -> [w1154 w1166 w1183 w1201]
              tunnel: [w1161 w1172 w1192 w1204] -> w901
              tunnel: [w1160 w1169 w1188 w1202] -> w900
              tunnel: [w1159 w1166 w1184 w1200] -> w899
              tunnel: [w1156 w1173 w1190 w1211] -> w898
              tunnel: [w1155 w1170 w1186 w1210] -> w897
              tunnel: [w1154 w1167 w1182 w1209] -> w896
              tunnel: w789 -> [w1158 w1164 w1181 w1208]
              tunnel: w788 -> [w1153 w1163 w1179 w1198]
              tunnel: [w1158 w1163 w1180 w1199] -> w787
              tunnel: [w1153 w1165 w1178 w1208] -> w786
              frame 0, Default {
              }
              frame 1 {
                n163 = Negate(x=w1177) -> (-x=w1176:i16)
                n164 = Negate(x=w1174) -> (-x=w1173:i16)
                n165 = Negate(x=w1164) -> (-x=w1165:i16)
                n166 = Negate(x=w1171) -> (-x=w1170:i16)
                n167 = Negate(x=w1168) -> (-x=w1167:i16)
              }
              frame 2 {
                n168 = Negate(x=w1197) -> (-x=w1196:i16)
                n169 = Negate(x=w1195) -> (-x=w1192:i16)
                n170 = Negate(x=w1191) -> (-x=w1190:i16)
                n171 = Negate(x=w1189) -> (-x=w1188:i16)
                n172 = Negate(x=w1187) -> (-x=w1186:i16)
                n173 = Negate(x=w1185) -> (-x=w1184:i16)
                n174 = Negate(x=w1183) -> (-x=w1182:i16)
                n175 = Negate(x=w1181) -> (-x=w1180:i16)
                n176 = Negate(x=w1179) -> (-x=w1178:i16)
                n177 = Negate(x=w1194) -> (-x=w1193:i16)
              }
              frame 3 {
                n178 = Negate(x=w1207) -> (-x=w1206:i16)
                n179 = Negate(x=w1205) -> (-x=w1204:i16)
                n180 = Negate(x=w1203) -> (-x=w1202:i16)
                n181 = Negate(x=w1201) -> (-x=w1200:i16)
                n182 = Negate(x=w1198) -> (-x=w1199:i16)
              }
            }
            n183 = Add(x=w717, y=w922) -> (x+y=w923:i32)
            n184 = xnode "Reinterpret Number"("x"=w734) -> ("y"=w733:fxp<+/-,16,17>)
            n185 = xnode "Reinterpret Number"("x"=w732) -> ("y"=w731:fxp<+/-,16,17>)
            n186 = xnode "Reinterpret Number"("x"=w726) -> ("y"=w725:fxp<+/-,16,17>)
            n187 = xnode "Reinterpret Number"("x"=w727) -> ("y"=w728:fxp<+/-,16,17>)
            n188 = xnode "Reinterpret Number"("x"=w730) -> ("y"=w729:fxp<+/-,16,17>)
            n189 = To Long Integer(number=w932) -> (32bit integer=w933:i32)
            n190 = xnode ("Memory Write")("Address"=w949, "Data"=w895, "Memory In"=w950) -> ()  [unwired: 1 out]
            n191 = To Long Integer(number=w895) -> (32bit integer=w945:i32)
            n192 = Square(x=w782) -> (x^2=w783:fxp<+,31,31>)
            n193 = Square(x=w781) -> (x^2=w784:fxp<+,31,31>)
            n194 = Subtract(x=w935, y=w933) -> (x-y=w916:i32)
            n195 = feedback #19() -> (w857:fxp<+,32,16>)  [unwired: 1 in]
            "amp3_out" <- w857
            n196 = feedback-in #19(w938) -> ()
            n197 = Add(x=w733, y=w837) -> (x+y=w808:fxp<+/-,32,18>)
            "phi0_full_out" <- w808
            n198 = Add(x=w731, y=w838) -> (x+y=w807:fxp<+/-,32,18>)
            "phi1_full_out" <- w807
            n199 = Add(x=w725, y=w812) -> (x+y=w806:fxp<+/-,32,18>)
            "phi2_full_out" <- w806
            n200 = Add(x=w728, y=w811) -> (x+y=w805:fxp<+/-,32,18>)
            "phi3_full_out" <- w805
            n201 = Add(x=w729, y=w762) -> (x+y=w761:fxp<+/-,32,18>)
            "phi4_full_out" <- w761
            n202 = xnode ("FIFO Write")("Element"=w747, "Timeout"=w750, "FIFO In"=w751) -> ()  [unwired: 2 out]
            n203 = Add(x=w783, y=w784) -> (x+y=w785:fxp<+,32,32>)
            n204 = Add(x=w715, y=w945) -> (x+y=w948:i32)
            n205 = xnode ("Memory Write")("Address"=w797, "Data"=w792, "Memory In"=w798) -> ()  [unwired: 1 out]
            n206 = To Long Integer(number=w792) -> (32bit integer=w795:i32)
            n207 = Square Root(x=w785) -> (sqrt(x)=w780:fxp<+,32,16>)
            n208 = xnode ("Memory Read")("Address"=w722, "Memory In"=w925) -> ("Data"=w920:i16)  [unwired: 1 out]
            n209 = To Word Integer(number=w716) -> (16bit integer=w912:i16)
            n210 = Add(x=w713, y=w795) -> (x+y=w796:i32)
            n211 = To Long Integer(number=w926) -> (32bit integer=w927:i32)
            n212 = feedback #20() -> (w776:fxp<+,32,16>)  [unwired: 1 in]
            "amp4_out" <- w776
            n213 = feedback-in #20(w780) -> ()
            n214 = xnode ("Memory Read")("Address"=w722, "Memory In"=w950) -> ("Data"=w943:i16)  [unwired: 1 out]
            n215 = To Word Integer(number=w714) -> (16bit integer=w913:i16)
            n216 = Subtract(x=w929, y=w927) -> (x-y=w915:i32)
            n217 = xnode ("Memory Read")("Address"=w722, "Memory In"=w798) -> ("Data"=w793:i16)  [unwired: 1 out]
            n218 = To Word Integer(number=w712) -> (16bit integer=w790:i16)
            n219 = To Long Integer(number=w920) -> (32bit integer=w921:i32)
            n220 = Subtract(x=w923, y=w921) -> (x-y=w914:i32)
            n221 = Build Array(w867, w866, w865, w864, w777) -> (w852:fxp<+/-,16,2>[])
            n222 = To Long Integer(number=w943) -> (32bit integer=w944:i32)
            n223 = Build Array(w860, w859, w858, w857, w776) -> (w853:fxp<+,32,16>[])
            n224 = Subtract(x=w948, y=w944) -> (x-y=w947:i32)
            n225 = Build Array(w903, w901, w900, w899, w787) -> (w894:i16[])
            n226 = To Long Integer(number=w793) -> (32bit integer=w794:i32)
            n227 = Build Array(w902, w898, w897, w896, w786) -> (w893:i16[])
            n228 = case shown="True" "reset_phi0" {
              tunnel: [w1120 i16 0] -> w850
              tunnel: w734 -> [w1120 _]
              frame False {
              }
              frame True {
              }
            }
            n229 = case shown="True" "reset_phi1" {
              tunnel: [w983 i16 0] -> w752
              tunnel: w732 -> [w983 _]
              frame False {
              }
              frame True {
              }
            }
            n230 = case shown="True" "reset_phi3" {
              tunnel: [w979 i16 0] -> w754
              tunnel: w727 -> [w979 _]
              frame False {
              }
              frame True {
              }
            }
            n231 = case shown="True" "reset_phi4" {
              tunnel: [w977 i16 0] -> w755
              tunnel: w730 -> [w977 _]
              frame False {
              }
              frame True {
              }
            }
            n232 = case shown="True" "reset_phi2" {
              tunnel: [w981 i16 0] -> w753
              tunnel: w726 -> [w981 _]
              frame False {
              }
              frame True {
              }
            }
            n233 = Subtract(x=w796, y=w794) -> (x-y=w791:i32)
            n234 = Build Array(w808, w807, w806, w805, w761) -> (w804:fxp<+/-,32,18>[])
            n235 = Add(x=u8 1, y=w709) -> (x+y=w968:u8)
            n236 = Build Array(w910, w911, w912, w913, w790) -> (w909:i16[])
          }
        }
      }
      n237 = while {
        stop <- FALSE stop-if-true
        n238 = flat-sequence {
          frame #0 {
            n239 = call "Loop Timer"("Count(uSec)"="trig_loop_timer (usec)") -> ()  [unwired: 1 out]
          }
          frame #1 {
            n240 = xnode "FPGA I/O Node"() -> ("Connector1/DIO22"=w30:bool)  [unwired: 1 in, 1 out]
            "DIO22" <- w30
            n241 = Not(x="block_config_trig") -> (.not. x?=w26:bool)
            n242 = Or(x=w30, y="manual_config_trig") -> (x .or. y?=w28:bool)
            n243 = call <instrlib>:"Detect Rising Edge.vi"("signal"=w28) -> ("edge detected"=w29:bool)  [unwired: 14 in]
            n244 = And(x=w29, y=w26) -> (x .and. y?=w23:bool)
            n245 = call <instrlib>:"Synchronous Latch.vi"("clear"="reset_config_trig", "set"=w23) -> ("out"=→"config_trig":bool)  [unwired: 9 in]
          }
        }
      }
      n246 = node-c288(w18) -> (w20:T1)
      n247 = while {
        stop <- FALSE stop-if-true
        # "3. Latch the Timekeeper's time when a new RT Time is detected. A Single Cycle Timed Loop is used to timestamp the RT Time update event as accurately as possible."
        # "4. Synchronize the FPGA Timekeeper to the RT Time by  giving the Timekeeper two timestamps associated to the RT Time update event:\n1. RT Time\n2. Timekeeper Time"
        n248 = node-c288() -> (w37:T1)  [unwired: 1 in]
        n249 = timed-loop {
          timing: w37 -> [_]
          timing-out: [_] -> w36
          shift-right: [w38] -> w34
          shift-left: "RT time (ns)" -> [w39]
          tunnel: [w41] -> w33
          stop <- w40 stop-if-true
          n250 = local read "RT time (ns)"() -> (w38:u64)
          n251 = Not Equal?(x=w38, y=w39) -> (x != y?=w40:bool)
          n252 = call "Get Time.vi"() -> ("time (ns)"=w41:u64)
        }
        n253 = node-c288(w36) -> ()
        n254 = call "Sync Time.vi"("FPGA Timekeeper time (ns)"=w33, "time reference time (ns)"=w34) -> ()
      }
      n255 = timed-loop {
        timing: w20 -> [_]
        timing-out: [_] -> w19
        shift-right: [w620] -> _
        shift-left: FALSE -> [w621]
        stop <- FALSE stop-if-true
        n256 = Not(x=w621) -> (.not. x?=w620:bool)
        n257 = xnode "FPGA I/O Node"("Connector1/DIO25"=w620, "TRIG0"="TRIG0") -> ()  [unwired: 2 in, 2 out]
      }
      n258 = node-c288(w19) -> ()
      n259 = while {
        shift-right: [w574] -> _
        shift-left: FALSE -> [w575]
        shift-right: [w572] -> _
        shift-left: _ -> [w570]
        stop <- FALSE stop-if-true
        n260 = flat-sequence {
          tunnel: w575 -> [w580]
          tunnel: [w579] -> w573
          tunnel: [w577] -> w571
          tunnel: w570 -> [w577]
          tunnel: w573 -> [w614]
          tunnel: [w614] -> w574
          tunnel: [w605] -> w572
          tunnel: w571 -> [_]
          frame #0 {
            n261 = Integer to Fixed-Point Cast(integer="loop timer (usec)") -> (fixed-point=→"loop time":fxp<+,32,32>)  [unwired: 1 in]
            n262 = Not(x=w580) -> (.not. x?=w579:bool)
            n263 = call "Loop Timer2"("Count(uSec)"="loop timer (usec)") -> ()  [unwired: 1 out]
          }
          frame #1 {
            w585 = refnum<k21> "power_hf"  # FIFO
            w589 = refnum<k21> "synch_line_hf"  # FIFO
            w609 = u16 0
            n264 = xnode "FPGA I/O Node"("Connector1/DIO24"=w614) -> ("Connector0/AI0"=w604:i16, "Connector0/AI1"=w597:i16, "Connector0/AI2"=w596:i16, "Connector0/AI3"=w595:i16, "Connector0/AI4"=w594:i16, "Connector0/AI7"=w583:i16, "Connector1/DIO23"=w587:bool)  [unwired: 8 in, 8 out]
            n265 = Build Array(w604, w597, w596, w595, w594) -> (w615:i16[])
            n266 = for {
              tunnel: w615 -> [w617] mode=indexing
              w618 = refnum<k21> "acq_data"  # FIFO
              n267 = xnode ("FIFO Write")("Element"=w617, "Timeout"=0, "FIFO In"=w618) -> ()  [unwired: 2 out]
            }
            n268 = feedback-in #21(w583) -> ()
            n269 = feedback #21() -> (w582:i16)  [unwired: 1 in]
            n270 = Number To Boolean Array(number=w594) -> (Boolean array=w598:bool[])
            n271 = Number To Boolean Array(number=w596) -> (Boolean array=w600:bool[])
            n272 = Number To Boolean Array(number=w595) -> (Boolean array=w599:bool[])
            n273 = Number To Boolean Array(number=w604) -> (Boolean array=w602:bool[])
            n274 = Number To Boolean Array(number=w597) -> (Boolean array=w601:bool[])
            n275 = feedback #22() -> (w586:bool)  [unwired: 1 in]
            n276 = feedback-in #22(w587) -> ()
            n277 = Boolean Array To Number(Boolean array=w598) -> (number=w590:u16)
            n278 = Boolean Array To Number(Boolean array=w600) -> (number=w592:u16)
            n279 = Boolean Array To Number(Boolean array=w599) -> (number=w591:u16)
            n280 = Boolean Array To Number(Boolean array=w602) -> (number=w603:u16)
            n281 = Boolean Array To Number(Boolean array=w601) -> (number=w593:u16)
            n282 = Join Numbers(hi=w603, lo=w593) -> ((hi.lo)=w613:u32)
            n283 = Join Numbers(hi=w592, lo=w591) -> ((hi.lo)=w612:u32)
            n284 = Join Numbers(hi=w590, lo=w609) -> ((hi.lo)=w611:u32)
            n285 = Join Numbers(hi=w609, lo=w609) -> ((hi.lo)=w610:u32)
            n286 = Join Numbers(hi=w613, lo=w612) -> ((hi.lo)=w608:u64)
            n287 = Join Numbers(hi=w611, lo=w610) -> ((hi.lo)=w607:u64)
            n288 = xnode ("FIFO Write")("Element"=w582, "Timeout"=0, "FIFO In"=w585) -> ()  [unwired: 2 out]
            n289 = xnode ("FIFO Write")("Element"=w586, "Timeout"=0, "FIFO In"=w589) -> ()  [unwired: 2 out]
            n290 = call "Get Time.vi"() -> ("time (ns)"=w606:u64)
            "time (ns)" <- w606
            n291 = Build Array(w608, w607, w606) -> (w605:u64[])
          }
        }
      }
      n292 = while {
        shift-right: [w498] -> _
        shift-left: i16 1 -> [w458]
        shift-right: [w490] -> _
        shift-left: fxp<+/-,64,32> 0.0 -> [w497]
        shift-right: [w489] -> _
        shift-left: fxp<+/-,64,32> 0.0 -> [w495]
        shift-right: [w480] -> _
        shift-left: fxp<+/-,64,32> 0.0 -> [w492]
        shift-right: [w476] -> _
        shift-left: i16 0 -> [w475]
        shift-right: [w462] -> _
        shift-left: _ -> [w460]
        shift-right: [w461] -> _
        shift-left: _ -> [w459]
        shift-right: [w452] -> _
        shift-left: fxp<+/-,64,32> 0.0 ("Numeric") -> [w451]
        stop <- FALSE stop-if-true
        w457 = refnum<k21> "power_hf"  # FIFO
        w471 = refnum<k21> "synch_line_hf"  # FIFO
        w487 = refnum<k21> "y_hf"  # FIFO
        w488 = refnum<k21> "x_hf"  # FIFO
        w493 = refnum<k21> "z_hf"  # FIFO
        w456 = i16 -1
        # "Take the (hf) sample at the digital \nport with the DAQ's sync output and \nadd to an I32 (convert to bool later). \nI32 gets written to a FIFO at the\ndownsample frequency"
        n293 = Equal To 0?(x=w458) -> (x = 0?=w486:bool)
        n294 = Equal To 0?(x=w458) -> (x = 0?=w465:bool)
        n295 = case shown="True" w486 {
          tunnel: w497 -> [w544 w557]
          tunnel: [w544 fxp<+/-,64,32> 0.0] -> w496
          tunnel: w495 -> [w543 w566]
          tunnel: [w543 fxp<+/-,64,36> 0.0] -> w494
          tunnel: w492 -> [w542 w565]
          tunnel: [w542 fxp<+/-,64,32> 0.0] -> w491
          tunnel: w475 -> [w541 w558]
          tunnel: [w541 i16 0] -> w474
          tunnel: w451 -> [w540 w549]
          tunnel: [w540 fxp<+/-,64,32> 0.0] -> w450
          frame False {
          }
          frame True {
            w547 = refnum<k21> "power_lf"  # FIFO
            w553 = refnum<k21> "y_lf"  # FIFO
            w554 = refnum<k21> "x_lf"  # FIFO
            w559 = refnum<k21> "synch_line_lf"  # FIFO
            w563 = refnum<k21> "z_lf"  # FIFO
            w562 = i16 0
            n296 = To Fixed-Point(number=w557) -> (fixed-point=w555:fxp<+/-,32,1>)  [unwired: 1 in]
            n297 = To Fixed-Point(number=w566) -> (fixed-point=w556:fxp<+/-,32,1>)  [unwired: 1 in]
            n298 = To Fixed-Point(number=w565) -> (fixed-point=w564:fxp<+/-,32,18>)  [unwired: 1 in]
            n299 = To Fixed-Point(number=w549) -> (fixed-point=w548:fxp<+/-,32,18>)  [unwired: 1 in]
            n300 = xnode "Reinterpret Number"("x"=w548) -> ("y"=w546:fxp<+/-,32,32>)
            n301 = xnode "Reinterpret Number"("x"=w555) -> ("y"=w552:fxp<+/-,32,32>)
            n302 = xnode "Reinterpret Number"("x"=w556) -> ("y"=w551:fxp<+/-,32,32>)
            n303 = xnode ("FIFO Write")("Element"=w558, "Timeout"=0, "FIFO In"=w559) -> ()  [unwired: 2 out]
            n304 = xnode ("FIFO Write")("Element"=w546, "Timeout"=0, "FIFO In"=w547) -> ()  [unwired: 2 out]
            n305 = xnode ("FIFO Write")("Element"=w552, "Timeout"=w562, "FIFO In"=w554) -> ()  [unwired: 2 out]
            n306 = xnode ("FIFO Write")("Element"=w551, "Timeout"=w562, "FIFO In"=w553) -> ()  [unwired: 2 out]
            n307 = xnode ("FIFO Write")("Element"=w564, "Timeout"=w562, "FIFO In"=w563) -> ()  [unwired: 2 out]
          }
        }
        n308 = case shown="True" w465 {
          tunnel: w460 -> [w503 w509]
          tunnel: [w503 fxp<+,64,32>[] [0.0, 0.0, 0.0, 0.0, 0.0]] -> w466
          tunnel: w459 -> [w502 w524]
          tunnel: [w502 fxp<+/-,64,32>[] [0.0, 0.0, 0.0, 0.0, 0.0]] -> w467
          frame False {
          }
          frame True {
            w506 = 0 ("Timeout")
            w507 = refnum<k21> "y_lf_2"  # FIFO
            w508 = refnum<k21> "x_lf_2"  # FIFO
            n309 = for {
              N: 5 -> [_]
              tunnel: w509 -> [w531] mode=indexing
              tunnel: w524 -> [w527] mode=indexing
              w526 = 0 ("Timeout")
              w529 = refnum<k21> "phi_lf"  # FIFO
              w532 = refnum<k21> "amp_lf"  # FIFO
              n310 = To Fixed-Point(number=w531) -> (fixed-point=w530:fxp<+,32,16>)  [unwired: 1 in]
              n311 = To Fixed-Point(number=w527) -> (fixed-point=w528:fxp<+/-,32,16>)  [unwired: 1 in]
              n312 = xnode ("FIFO Write")("Element"=w530, "Timeout"=w526, "FIFO In"=w532) -> ()  [unwired: 2 out]
              n313 = xnode ("FIFO Write")("Element"=w528, "Timeout"=w526, "FIFO In"=w529) -> ()  [unwired: 2 out]
            }
            n314 = Index Array(array=w509) -> (element #1=w518:fxp<+,64,32>, element #2=w520:fxp<+,64,32>, element #3=w519:fxp<+,64,32>, element #4=w521:fxp<+,64,32>)  [unwired: 4 in]
            n315 = Add(x=w518, y=w520) -> (x+y=w514:fxp<+,64,32>)
            n316 = Add(x=w519, y=w521) -> (x+y=w515:fxp<+,64,32>)
            n317 = Add(x=w518, y=w519) -> (x+y=w517:fxp<+,64,32>)
            n318 = Add(x=w520, y=w521) -> (x+y=w516:fxp<+,64,32>)
            n319 = Subtract(x=w514, y=w515) -> (x-y=w511:fxp<+/-,64,32>)
            n320 = Add(x=w514, y=w515) -> (x+y=w510:fxp<+,64,32>)
            n321 = Subtract(x=w517, y=w516) -> (x-y=w513:fxp<+/-,64,32>)
            n322 = Add(x=w517, y=w516) -> (x+y=w512:fxp<+,64,32>)
            n323 = Divide(x=w513, y=w512) -> (x/y=w505:fxp<+/-,64,32>)
            n324 = Divide(x=w511, y=w510) -> (x/y=w504:fxp<+/-,64,32>)
            n325 = xnode ("FIFO Write")("Element"=w504, "Timeout"=w506, "FIFO In"=w508) -> ()  [unwired: 2 out]
            n326 = xnode ("FIFO Write")("Element"=w505, "Timeout"=w506, "FIFO In"=w507) -> ()  [unwired: 2 out]
          }
        }
        n327 = for {
          N: 5 -> [_]
          tunnel: [w533] -> w464 mode=indexing
          tunnel: [w534] -> w463 mode=indexing
          w538 = refnum<k21> "phi_hf"  # FIFO
          w537 = i16 -1
          w539 = refnum<k21> "amp_hf"  # FIFO
          n328 = xnode ("FIFO Read")("Timeout"=w537, "FIFO In"=w539) -> ("Element"=w536:fxp<+,32,16>)  [unwired: 2 out]
          n329 = xnode ("FIFO Read")("Timeout"=w537, "FIFO In"=w538) -> ("Element"=w535:fxp<+/-,32,18>)  [unwired: 2 out]
          n330 = xnode "Reinterpret Number"("x"=w536) -> ("y"=w533:fxp<+/-,32,9>)
          n331 = xnode "Reinterpret Number"("x"=w535) -> ("y"=w534:fxp<+/-,32,11>)
        }
        n332 = xnode ("FIFO Read")("Timeout"=w456, "FIFO In"=w488) -> ("Element"=w485:fxp<+/-,64,32>)  [unwired: 2 out]
        n333 = xnode ("FIFO Read")("Timeout"=w456, "FIFO In"=w487) -> ("Element"=w483:fxp<+/-,64,32>)  [unwired: 2 out]
        n334 = xnode ("FIFO Read")("Timeout"=w456, "FIFO In"=w493) -> ("Element"=w479:fxp<+/-,32,18>)  [unwired: 2 out]
        n335 = xnode ("FIFO Read")("Timeout"=w456, "FIFO In"=w457) -> ("Element"=w455:i16)  [unwired: 2 out]
        n336 = Increment(x=w458) -> (x+1=w500:i16)
        n337 = Quotient & Remainder(x=w500, y="downsamp_num") -> (x-y*floor(x/y)=w498:i16)  [unwired: 1 out]
        n338 = To Fixed-Point(number=w455) -> (fixed-point=w454:fxp<+/-,64,32>)  [unwired: 1 in]
        n339 = To Fixed-Point(number=w479) -> (fixed-point=w478:fxp<+/-,64,32>)  [unwired: 1 in]
        n340 = xnode "Reinterpret Number"("x"=w485) -> ("y"=w484:fxp<+/-,64,25>)
        n341 = xnode "Reinterpret Number"("x"=w483) -> ("y"=w482:fxp<+/-,64,25>)
        n342 = xnode "Reinterpret Number"("x"=w478) -> ("y"=w481:fxp<+/-,64,25>)
        n343 = xnode "Reinterpret Number"("x"=w454) -> ("y"=w453:fxp<+/-,64,25>)
        n344 = xnode ("FIFO Read")("Timeout"=-1, "FIFO In"=w471) -> ("Element"=w470:bool)  [unwired: 2 out]
        n345 = Select(t=i16 1, s=w470, f=i16 -1) -> (s? t:f=w477:i16)
        n346 = Add(x=w477, y=w474) -> (x+y=w476:i16)
        n347 = Add(x=w484, y=w496) -> (x+y=w490:fxp<+/-,64,32>)
        n348 = Add(x=w464, y=w466) -> (x+y=w462:fxp<+,64,32>[])
        n349 = Add(x=w482, y=w494) -> (x+y=w489:fxp<+/-,64,32>)
        n350 = Add(x=w463, y=w467) -> (x+y=w461:fxp<+/-,64,32>[])
        n351 = Add(x=w481, y=w491) -> (x+y=w480:fxp<+/-,64,32>)
        n352 = Add(x=w453, y=w450) -> (x+y=w452:fxp<+/-,64,32>)
      }
      n353 = while {
        shift-right: [w152] -> _
        shift-left: _ -> [w281]
        shift-right: [w278] -> _
        shift-left: TRUE -> [w273]
        shift-right: [w238] -> _
        shift-left: _ -> [w241]
        shift-right: [w168] -> _
        shift-left: _ -> [w150]
        shift-right: [w149] -> _
        shift-left: _ -> [w148]
        shift-right: [w110] -> _
        shift-left: _ -> [w109]
        shift-right: [w47] -> _
        shift-left: _ -> [w46]
        stop <- FALSE stop-if-true
        w118 = refnum<k21> "power_lf"  # FIFO
        w182 = refnum<k21> "y_lf_2"  # FIFO
        w181 = i16 -1
        w183 = refnum<k21> "x_lf_2"  # FIFO
        w187 = refnum<k21> "y_lf"  # FIFO
        w188 = refnum<k21> "x_lf"  # FIFO
        w192 = refnum<k21> "synch_line_lf"  # FIFO
        w285 = refnum<k21> "z_lf"  # FIFO
        w286 = i16 -1
        # "internal injection frequency relative \nto top level clock"
        # "Compute derivative as the \ndifference between neighboring \nsamples, then average two \nsamples with a sum and bitshift\nright by one (33,33)->(33,32) to \ndivide by 2"
        n354 = xnode ("FIFO Read")("Timeout"=w181, "FIFO In"=w182) -> ("Element"=w177:fxp<+/-,64,32>)  [unwired: 2 out]
        n355 = xnode ("FIFO Read")("Timeout"=w286, "FIFO In"=w188) -> ("Element"=w190:fxp<+/-,32,32>)  [unwired: 2 out]
        n356 = xnode ("FIFO Read")("Timeout"=w286, "FIFO In"=w187) -> ("Element"=w189:fxp<+/-,32,32>)  [unwired: 2 out]
        n357 = xnode ("FIFO Read")("Timeout"=w181, "FIFO In"=w183) -> ("Element"=w180:fxp<+/-,64,32>)  [unwired: 2 out]
        n358 = xnode ("FIFO Read")("Timeout"=w286, "FIFO In"=w285) -> ("Element"=w276:fxp<+/-,32,18>)  [unwired: 2 out]
        n359 = xnode ("FIFO Read")("Timeout"=0, "FIFO In"=w118) -> ("Element"=w115:fxp<+/-,32,32>)  [unwired: 2 out]
        n360 = xnode ("FIFO Read")("Timeout"=-1, "FIFO In"=w192) -> ("Element"=w191:i32)  [unwired: 2 out]
        n361 = To Fixed-Point(number=w177) -> (fixed-point=w178:fxp<+/-,32,1>)  [unwired: 1 in]
        n362 = To Fixed-Point(number=w180) -> (fixed-point=w179:fxp<+/-,32,1>)  [unwired: 1 in]
        n363 = xnode "Reinterpret Number"("x"=w276) -> ("y"=w212:fxp<+/-,32,32>)
        n364 = for {
          N: 5 -> [_]
          tunnel: [w347] -> w146 mode=indexing
          tunnel: [w343] -> w130 mode=indexing
          w352 = refnum<k21> "phi_lf"  # FIFO
          w351 = -1 ("Timeout")
          w353 = refnum<k21> "amp_lf"  # FIFO
          n365 = xnode ("FIFO Read")("Timeout"=w351, "FIFO In"=w353) -> ("Element"=w350:fxp<+,32,16>)  [unwired: 2 out]
          n366 = xnode ("FIFO Read")("Timeout"=w351, "FIFO In"=w352) -> ("Element"=w348:fxp<+/-,32,16>)  [unwired: 2 out]
          n367 = xnode "Reinterpret Number"("x"=w350) -> ("y"=w344:fxp<+,32,32>)
          n368 = xnode "Reinterpret Number"("x"=w348) -> ("y"=w349:fxp<+/-,32,32>)
          n369 = To Unsigned Long Integer(number=w344) -> (unsigned 32bit integer=w345:u32)
          n370 = To Long Integer(number=w349) -> (32bit integer=w347:i32)
          n371 = Number To Boolean Array(number=w345) -> (Boolean array=w346:bool[])
          n372 = Boolean Array To Number(Boolean array=w346) -> (number=w343:i32)
        }
        n373 = xnode "Reinterpret Number"("x"=w178) -> ("y"=w173:fxp<+/-,32,32>)
        n374 = xnode "Reinterpret Number"("x"=w179) -> ("y"=w175:fxp<+/-,32,32>)
        n375 = Less Than 0?(x=w115) -> (x < 0?=w116:bool)
        n376 = Less Than 0?(x=w189) -> (x < 0?=w216:bool)
        n377 = Less Than 0?(x=w190) -> (x < 0?=w217:bool)
        n378 = Less Than 0?(x=w212) -> (x < 0?=w215:bool)
        n379 = Less Than 0?(x=w175) -> (x < 0?=w176:bool)
        n380 = Less Than 0?(x=w173) -> (x < 0?=w174:bool)
        n381 = case shown="False" w116 {
          tunnel: "pow_bitshift" -> [w332 w337]
          tunnel: [w330 w333] -> w51
          tunnel: w115 -> [w331 w336]
          frame False {
            n382 = Logical Shift(y=w332, x=w331) -> (x << y=w330:fxp<+/-,32,32>)
          }
          frame True {
            n383 = Negate(x=w336) -> (-x=w335:fxp<+/-,32,32>)
            n384 = Logical Shift(y=w337, x=w335) -> (x << y=w334:fxp<+/-,32,32>)
            n385 = Negate(x=w334) -> (-x=w333:fxp<+/-,32,32>)
          }
        }
        n386 = To Long Integer(number=w51) -> (32bit integer=→"pow_shifted":i32)
        n387 = case shown="True" w217 {
          tunnel: "xy_bitshift" -> [w439 w444]
          tunnel: [w437 w440] -> w157
          tunnel: w190 -> [w438 w443]
          frame False {
            n388 = Logical Shift(y=w439, x=w438) -> (x << y=w437:fxp<+/-,32,32>)
          }
          frame True {
            n389 = Negate(x=w443) -> (-x=w442:fxp<+/-,32,32>)
            n390 = Logical Shift(y=w444, x=w442) -> (x << y=w441:fxp<+/-,32,32>)
            n391 = Negate(x=w441) -> (-x=w440:fxp<+/-,32,32>)
          }
        }
        n392 = case shown="True" w216 {
          tunnel: "xy_bitshift" -> [w431 w436]
          tunnel: [w429 w432] -> w156
          tunnel: w189 -> [w430 w435]
          frame False {
            n393 = Logical Shift(y=w431, x=w430) -> (x << y=w429:fxp<+/-,32,32>)
          }
          frame True {
            n394 = Negate(x=w435) -> (-x=w434:fxp<+/-,32,32>)
            n395 = Logical Shift(y=w436, x=w434) -> (x << y=w433:fxp<+/-,32,32>)
            n396 = Negate(x=w433) -> (-x=w432:fxp<+/-,32,32>)
          }
        }
        n397 = case shown="False" w215 {
          tunnel: "z_bitshift" -> [w423 w428]
          tunnel: [w421 w424] -> w151
          tunnel: w212 -> [w422 w427]
          frame False {
            n398 = Logical Shift(y=w423, x=w422) -> (x << y=w421:fxp<+/-,32,32>)
          }
          frame True {
            n399 = Negate(x=w427) -> (-x=w426:fxp<+/-,32,32>)
            n400 = Logical Shift(y=w428, x=w426) -> (x << y=w425:fxp<+/-,32,32>)
            n401 = Negate(x=w425) -> (-x=w424:fxp<+/-,32,32>)
          }
        }
        n402 = case shown="True" w176 {
          tunnel: "xy2_bitshift" -> [w375 w380]
          tunnel: [w373 w376] -> w159
          tunnel: w175 -> [w374 w379]
          frame False {
            n403 = Logical Shift(y=w375, x=w374) -> (x << y=w373:fxp<+/-,32,32>)
          }
          frame True {
            n404 = Negate(x=w379) -> (-x=w378:fxp<+/-,32,32>)
            n405 = Logical Shift(y=w380, x=w378) -> (x << y=w377:fxp<+/-,32,32>)
            n406 = Negate(x=w377) -> (-x=w376:fxp<+/-,32,32>)
          }
        }
        n407 = case shown="True" w174 {
          tunnel: "xy2_bitshift" -> [w367 w372]
          tunnel: [w365 w368] -> w158
          tunnel: w173 -> [w366 w371]
          frame False {
            n408 = Logical Shift(y=w367, x=w366) -> (x << y=w365:fxp<+/-,32,32>)
          }
          frame True {
            n409 = Negate(x=w371) -> (-x=w370:fxp<+/-,32,32>)
            n410 = Logical Shift(y=w372, x=w370) -> (x << y=w369:fxp<+/-,32,32>)
            n411 = Negate(x=w369) -> (-x=w368:fxp<+/-,32,32>)
          }
        }
        n412 = feedback #23() -> (w100:fxp<+/-,32,32>)  [unwired: 1 in]
        n413 = Build Array(w159, w158, w157, w156, w151) -> (w155:fxp<+/-,32,32>[])
        n414 = case shown="True" "downsample->xyz" {
          tunnel: w159 -> [_ w364]
          tunnel: w158 -> [_ w363]
          tunnel: w157 -> [w362 _]
          tunnel: w156 -> [w361 _]
          tunnel: [w362 w364] -> w170
          tunnel: [w361 w363] -> w169
          frame False {
          }
          frame True {
          }
        }
        n415 = Index Array(array=w146) -> (element #1=w135:i32, element #2=w134:i32, element #3=w133:i32, element #4=w132:i32, element #5=w131:i32)  [unwired: 5 in]
        n416 = Index Array(array=w130) -> (element #1=w139:i32, element #2=w138:i32, element #3=w137:i32, element #4=w136:i32, element #5=w101:i32)  [unwired: 5 in]
        "amp4_lf" <- w101
        n417 = To Long Integer(number=w155) -> (32bit integer=w153:i32[])
        n418 = feedback #24() -> (w98:fxp<+/-,32,32>)  [unwired: 1 in]
        n419 = for {
          tunnel: w148 -> [w342] mode=indexing
          w340 = refnum<k21> "host_amp-phi"  # FIFO
          n420 = xnode ("FIFO Write")("Element"=w342, "Timeout"=0, "FIFO In"=w340) -> ()  [unwired: 2 out]
        }
        n421 = local read "time (ns)"() -> (w129:u64)
        n422 = To Long Integer(number=w170) -> (32bit integer=→"x_shifted":i32)
        n423 = To Long Integer(number=w169) -> (32bit integer=→"y_shifted":i32)
        n424 = To Long Integer(number=w151) -> (32bit integer=→"z_shifted":i32)
        n425 = Split Number(x=w129) -> (hi(x)=w143:u32, lo(x)=w142:u32)
        n426 = Subtract(x=w151, y="z_set_user") -> (x-y=w242:fxp<+/-,32,32>)
        n427 = feedback #25() -> (w265:fxp<+/-,32,32>)  [unwired: 1 in]
        n428 = feedback-in #25(w169) -> ()
        n429 = feedback #26() -> (w274:fxp<+/-,32,32>)  [unwired: 1 in]
        n430 = feedback-in #26(w170) -> ()
        n431 = feedback #27() -> (w256:fxp<+/-,32,32>)  [unwired: 1 in]
        n432 = feedback-in #27(w242) -> ()
        n433 = Number To Boolean Array(number=w143) -> (Boolean array=w144:bool[])
        n434 = Number To Boolean Array(number=w142) -> (Boolean array=w145:bool[])
        n435 = Select(t=FALSE, s=w273, f=TRUE) -> (s? t:f=w278:bool)
        n436 = Subtract(x=w169, y=w265) -> (x-y=w264:fxp<+/-,32,32>)
        n437 = Subtract(x=w170, y=w274) -> (x-y=w272:fxp<+/-,32,32>)
        n438 = Subtract(x=w242, y=w256) -> (x-y=w255:fxp<+/-,32,32>)
        n439 = Boolean Array To Number(Boolean array=w144) -> (number=w141:i32)
        n440 = Boolean Array To Number(Boolean array=w145) -> (number=w140:i32)
        n441 = feedback #28() -> (w263:fxp<+/-,32,32>)  [unwired: 1 in]
        n442 = feedback-in #28(w264) -> ()
        n443 = feedback #29() -> (w271:fxp<+/-,32,32>)  [unwired: 1 in]
        n444 = feedback-in #29(w272) -> ()
        n445 = feedback #30() -> (w254:fxp<+/-,32,32>)  [unwired: 1 in]
        n446 = feedback-in #30(w255) -> ()
        n447 = Build Array(w139, w138, w137, w136, w101, w135, w134, w133, w132, w131, w141, w140) -> (w149:i32[])
        n448 = Add(x=w264, y=w263) -> (x+y=w262:fxp<+/-,33,33>)
        n449 = Add(x=w272, y=w271) -> (x+y=w270:fxp<+/-,33,33>)
        n450 = Add(x=w255, y=w254) -> (x+y=w253:fxp<+/-,33,33>)
        n451 = Add(x=w242, y=w241) -> (x+y=w239:fxp<+/-,64,64>)
        n452 = xnode "Reinterpret Number"("x"=w262) -> ("y"=w261:fxp<+/-,33,32>)
        n453 = xnode "Reinterpret Number"("x"=w270) -> ("y"=w269:fxp<+/-,33,32>)
        n454 = xnode "Reinterpret Number"("x"=w253) -> ("y"=w252:fxp<+/-,33,32>)
        n455 = for {
          tunnel: w281 -> [w449] mode=indexing
          w447 = refnum<k21> "host_xyz"  # FIFO
          n456 = xnode ("FIFO Write")("Element"=w449, "Timeout"=i16 0, "FIFO In"=w447) -> ()  [unwired: 2 out]
        }
        n457 = To Fixed-Point(number=w269) -> (fixed-point=w268:fxp<+/-,32,32>)  [unwired: 1 in]
        n458 = To Fixed-Point(number=w261) -> (fixed-point=w260:fxp<+/-,32,32>)  [unwired: 1 in]
        n459 = To Fixed-Point(number=w252) -> (fixed-point=w251:fxp<+/-,32,32>)  [unwired: 1 in]
        n460 = To Fixed-Point(number=w239) -> (fixed-point=w240:fxp<+/-,32,32>)  [unwired: 1 in]
        n461 = Multiply(x="x_dg", y=w268) -> (x*y=w266:fxp<+/-,64,48>)
        n462 = Multiply(x="y_dg", y=w260) -> (x*y=w258:fxp<+/-,64,48>)
        n463 = Multiply(x="z_dg", y=w251) -> (x*y=w249:fxp<+/-,64,48>)
        n464 = Multiply(x="z_pg", y=w242) -> (x*y=w244:fxp<+/-,64,48>)
        n465 = Multiply(x="z_ig", y=w240) -> (x*y=w236:fxp<+/-,64,48>)
        n466 = xnode "Reinterpret Number"("x"=w266) -> ("y"=w203:fxp<+/-,64,64>)
        n467 = xnode "Reinterpret Number"("x"=w258) -> ("y"=w202:fxp<+/-,64,64>)
        n468 = xnode "Reinterpret Number"("x"=w249) -> ("y"=w205:fxp<+/-,64,64>)
        n469 = xnode "Reinterpret Number"("x"=w244) -> ("y"=w207:fxp<+/-,64,64>)
        n470 = xnode "Reinterpret Number"("x"=w236) -> ("y"=w210:fxp<+/-,64,64>)
        n471 = Less Than 0?(x=w203) -> (x < 0?=w199:bool)
        n472 = Less Than 0?(x=w202) -> (x < 0?=w198:bool)
        n473 = Less Than 0?(x=w205) -> (x < 0?=w206:bool)
        n474 = Less Than 0?(x=w207) -> (x < 0?=w208:bool)
        n475 = Less Than 0?(x=w210) -> (x < 0?=w209:bool)
        n476 = case shown="True" w199 {
          tunnel: "xy_fb_bitshift" -> [w415 w420]
          tunnel: [w413 w416] -> w201
          tunnel: w203 -> [w414 w419]
          frame False {
            n477 = Logical Shift(y=w415, x=w414) -> (x << y=w413:fxp<+/-,64,64>)
          }
          frame True {
            n478 = Negate(x=w419) -> (-x=w418:fxp<+/-,64,64>)
            n479 = Logical Shift(y=w420, x=w418) -> (x << y=w417:fxp<+/-,64,64>)
            n480 = Negate(x=w417) -> (-x=w416:fxp<+/-,64,64>)
          }
        }
        n481 = case shown="True" w198 {
          tunnel: "xy_fb_bitshift" -> [w407 w412]
          tunnel: [w405 w408] -> w200
          tunnel: w202 -> [w406 w411]
          frame False {
            n482 = Logical Shift(y=w407, x=w406) -> (x << y=w405:fxp<+/-,64,64>)
          }
          frame True {
            n483 = Negate(x=w411) -> (-x=w410:fxp<+/-,64,64>)
            n484 = Logical Shift(y=w412, x=w410) -> (x << y=w409:fxp<+/-,64,64>)
            n485 = Negate(x=w409) -> (-x=w408:fxp<+/-,64,64>)
          }
        }
        n486 = case shown="True" w206 {
          tunnel: "z_fb_bitshift" -> [w399 w404]
          tunnel: [w397 w400] -> w67
          tunnel: w205 -> [w398 w403]
          frame False {
            n487 = Logical Shift(y=w399, x=w398) -> (x << y=w397:fxp<+/-,64,64>)
          }
          frame True {
            n488 = Negate(x=w403) -> (-x=w402:fxp<+/-,64,64>)
            n489 = Logical Shift(y=w404, x=w402) -> (x << y=w401:fxp<+/-,64,64>)
            n490 = Negate(x=w401) -> (-x=w400:fxp<+/-,64,64>)
          }
        }
        n491 = case shown="True" w208 {
          tunnel: "z_fb_bitshift" -> [w391 w396]
          tunnel: [w389 w392] -> w66
          tunnel: w207 -> [w390 w395]
          frame False {
            n492 = Logical Shift(y=w391, x=w390) -> (x << y=w389:fxp<+/-,64,64>)
          }
          frame True {
            n493 = Negate(x=w395) -> (-x=w394:fxp<+/-,64,64>)
            n494 = Logical Shift(y=w396, x=w394) -> (x << y=w393:fxp<+/-,64,64>)
            n495 = Negate(x=w393) -> (-x=w392:fxp<+/-,64,64>)
          }
        }
        n496 = case shown="True" w209 {
          tunnel: "z_fb_bitshift" -> [w383 w388]
          tunnel: [w381 w384] -> w65
          tunnel: w210 -> [w382 w387]
          frame False {
            n497 = Logical Shift(y=w383, x=w382) -> (x << y=w381:fxp<+/-,64,64>)
          }
          frame True {
            n498 = Negate(x=w387) -> (-x=w386:fxp<+/-,64,64>)
            n499 = Logical Shift(y=w388, x=w386) -> (x << y=w385:fxp<+/-,64,64>)
            n500 = Negate(x=w385) -> (-x=w384:fxp<+/-,64,64>)
          }
        }
        n501 = for {
          tunnel: w46 -> [w288] mode=indexing
          w290 = refnum<k21> "host_pow"  # FIFO
          n502 = xnode "FIFO Write"("Element"=w288, "Timeout"=0, "FIFO In"=w290) -> ()  [unwired: 2 out]
        }
        n503 = call "Sine Wave Generator"("frequency (periods/tick)"="z_internal_inject_freq") -> ("sine out"=w127:i16)  [unwired: 14 in]
        n504 = Quotient & Remainder(x=w127, y="z_internal_inject_scale") -> (floor(x/y)=w124:i16)  [unwired: 1 out]
        n505 = To Word Integer(number=w67) -> (16bit integer=w248:i16)
        n506 = To Word Integer(number=w66) -> (16bit integer=w247:i16)
        n507 = To Word Integer(number=w65) -> (16bit integer=w246:i16)
        n508 = Add(x=w67, y=w66) -> (x+y=w64:fxp<+/-,64,64>)
        n509 = Add(x=w64, y=w65) -> (x+y=w63:fxp<+/-,64,64>)
        n510 = To Fixed-Point(number=w63) -> (fixed-point=w53:fxp<+/-,32,32>)  [unwired: 1 in]
        n511 = Greater?(x=w53, y="delta_pow_set_ulim") -> (0:w105:bool)
        n512 = Select(t="delta_pow_set_ulim", s=w105, f=w53) -> (s? t:f=w103:fxp<+/-,32,32>)
        n513 = Less?(x=w103, y="delta_pow_set_llim") -> (x < y?=w104:bool)
        n514 = Select(t="delta_pow_set_llim", s=w104, f=w103) -> (s? t:f=w59:fxp<+/-,32,32>)
        "delta_pow_set" <- w59
        n515 = case shown="True" "fb_on_pow_set" {
          tunnel: w59 -> [_ w294]
          tunnel: [w291 w293] -> w57
          tunnel: "pow_set_user" -> [w291 w292]
          frame False {
          }
          frame True {
            n516 = Add(x=w294, y=w292) -> (x+y=w293:fxp<+/-,33,33>)
          }
        }
        "pow_set_actual" <- w57
        n517 = Subtract(x=w51, y=w57) -> (x-y=w77:fxp<+/-,32,32>)
        n518 = feedback-in #23(w77) -> ()
        n519 = Add(x=w77, y=w109) -> (x+y=w108:fxp<+/-,64,64>)
        n520 = Subtract(x=w77, y=w100) -> (x-y=w99:fxp<+/-,32,32>)
        n521 = feedback-in #24(w99) -> ()
        n522 = Add(x=w99, y=w98) -> (x+y=w97:fxp<+/-,33,33>)
        n523 = xnode "Reinterpret Number"("x"=w97) -> ("y"=w96:fxp<+/-,33,32>)
        n524 = To Fixed-Point(number=w108) -> (fixed-point=w112:fxp<+/-,32,32>)  [unwired: 1 in]
        n525 = To Fixed-Point(number=w96) -> (fixed-point=w95:fxp<+/-,32,32>)  [unwired: 1 in]
        n526 = Multiply(x="pow_ig", y=w112) -> (x*y=w107:fxp<+/-,64,48>)
        n527 = Multiply(x="pow_dg", y=w95) -> (x*y=w93:fxp<+/-,64,48>)
        n528 = Multiply(x="pow_pg", y=w77) -> (x*y=w91:fxp<+/-,64,48>)
        n529 = xnode "Reinterpret Number"("x"=w93) -> ("y"=w80:fxp<+/-,64,64>)
        n530 = xnode "Reinterpret Number"("x"=w91) -> ("y"=w81:fxp<+/-,64,64>)
        n531 = xnode "Reinterpret Number"("x"=w107) -> ("y"=w78:fxp<+/-,64,64>)
        n532 = Less Than 0?(x=w80) -> (x < 0?=w84:bool)
        n533 = Less Than 0?(x=w81) -> (x < 0?=w85:bool)
        n534 = Less Than 0?(x=w78) -> (x < 0?=w86:bool)
        n535 = case shown="True" w84 {
          tunnel: "pow_fb_bitshift" -> [w322 w327]
          tunnel: [w320 w323] -> w87
          tunnel: w80 -> [w321 w326]
          frame False {
            n536 = Logical Shift(y=w322, x=w321) -> (x << y=w320:fxp<+/-,64,64>)
          }
          frame True {
            n537 = Negate(x=w326) -> (-x=w325:fxp<+/-,64,64>)
            n538 = Logical Shift(y=w327, x=w325) -> (x << y=w324:fxp<+/-,64,64>)
            n539 = Negate(x=w324) -> (-x=w323:fxp<+/-,64,64>)
          }
        }
        n540 = case shown="True" w85 {
          tunnel: "pow_fb_bitshift" -> [w314 w319]
          tunnel: [w312 w315] -> w88
          tunnel: w81 -> [w313 w318]
          frame False {
            n541 = Logical Shift(y=w314, x=w313) -> (x << y=w312:fxp<+/-,64,64>)
          }
          frame True {
            n542 = Negate(x=w318) -> (-x=w317:fxp<+/-,64,64>)
            n543 = Logical Shift(y=w319, x=w317) -> (x << y=w316:fxp<+/-,64,64>)
            n544 = Negate(x=w316) -> (-x=w315:fxp<+/-,64,64>)
          }
        }
        n545 = case shown="True" w86 {
          tunnel: "pow_fb_bitshift" -> [w306 w311]
          tunnel: [w304 w307] -> w89
          tunnel: w78 -> [w305 w310]
          frame False {
            n546 = Logical Shift(y=w306, x=w305) -> (x << y=w304:fxp<+/-,64,64>)
          }
          frame True {
            n547 = Negate(x=w310) -> (-x=w309:fxp<+/-,64,64>)
            n548 = Logical Shift(y=w311, x=w309) -> (x << y=w308:fxp<+/-,64,64>)
            n549 = Negate(x=w308) -> (-x=w307:fxp<+/-,64,64>)
          }
        }
        n550 = To Word Integer(number=w87) -> (16bit integer=w83:i16)
        n551 = To Word Integer(number=w88) -> (16bit integer=w90:i16)
        n552 = To Word Integer(number=w89) -> (16bit integer=w82:i16)
        n553 = Compound Arithmetic op=ADD(w83, w90, w82) -> (w71:i16)
        n554 = Greater?(x=w71, y="pow_upper_lim") -> (0:w76:bool)
        n555 = Select(t="pow_upper_lim", s=w76, f=w71) -> (s? t:f=w73:i16)
        n556 = Less?(x=w73, y="pow_lower_lim") -> (x < y?=w74:bool)
        n557 = Select(t="pow_lower_lim", s=w74, f=w73) -> (s? t:f=w55:i16)
        n558 = To Word Integer(number=w201) -> (16bit integer=w234:i16)
        n559 = To Word Integer(number=w200) -> (16bit integer=w224:i16)
        n560 = Compound Arithmetic op=ADD(w248, w247, w246) -> (w218:i16)
        n561 = case shown="False" "add_sin" {
          tunnel: w124 -> [_ w339]
          tunnel: [i16 0 w339] -> w123
          frame False {
          }
          frame True {
          }
        }
        n562 = Greater?(x=w234, y="x_upper_lim") -> (0:w235:bool)
        n563 = Greater?(x=w224, y="y_upper_lim") -> (0:w229:bool)
        n564 = Add(x="pow_dc_offset", y=w55) -> (x+y=w54:i16)
        n565 = Greater?(x=w218, y="z_upper_lim") -> (0:w223:bool)
        n566 = Select(t="x_upper_lim", s=w235, f=w234) -> (s? t:f=w231:i16)
        n567 = Select(t="y_upper_lim", s=w229, f=w224) -> (s? t:f=w226:i16)
        n568 = Select(t="z_upper_lim", s=w223, f=w218) -> (s? t:f=w220:i16)
        n569 = case shown="True" "inject_sigs" {
          tunnel: [i16 0 ("x+y") w359] -> w163
          tunnel: [i16 0 ("x+y") w358] -> w162
          tunnel: [i16 0 ("x+y") w357] -> w122
          tunnel: w150 -> [_ w360]
          frame False {
          }
          frame True {
            n570 = Index Array(array=w360) -> (element #1=w359:i16, element #2=w358:i16, element #3=w357:i16)  [unwired: 3 in]
          }
        }
        n571 = Less?(x=w231, y="x_lower_lim") -> (x < y?=w232:bool)
        n572 = Less?(x=w226, y="y_lower_lim") -> (x < y?=w227:bool)
        n573 = Less?(x=w220, y="z_lower_lim") -> (x < y?=w221:bool)
        n574 = Select(t="x_lower_lim", s=w232, f=w231) -> (s? t:f=w186:i16)
        "x_fb_i16" <- w186
        n575 = Select(t="y_lower_lim", s=w227, f=w226) -> (s? t:f=w185:i16)
        "y_fb_i16" <- w185
        n576 = Select(t="z_lower_lim", s=w221, f=w220) -> (s? t:f=w184:i16)
        "z_fb_i16" <- w184
        n577 = case shown="True" "reset_pow_accum" {
          tunnel: w108 -> [w328 _]
          tunnel: [w328 fxp<+/-,64,64> 0.0] -> w110
          frame False {
          }
          frame True {
          }
        }
        n578 = case shown="True" "reset_z_accum" {
          tunnel: w239 -> [w445 _]
          tunnel: [w445 fxp<+/-,64,64> 0.0] -> w238
          frame False {
          }
          frame True {
          }
        }
        n579 = Add(x="x_dc_offset", y=w186) -> (x+y=w166:i16)
        n580 = Add(x="y_dc_offset", y=w185) -> (x+y=w164:i16)
        n581 = Add(x="z_dc_offset", y=w184) -> (x+y=w165:i16)
        n582 = Add(x=w122, y=w123) -> (x+y=w121:i16)
        n583 = Split Number(x=w129) -> (hi(x)=w197:u32, lo(x)=w194:u32)
        n584 = Add(x=w162, y=w164) -> (x+y=w161:i16)
        n585 = Add(x=w121, y=w165) -> (x+y=w69:i16)
        n586 = Add(x=w163, y=w166) -> (x+y=w160:i16)
        n587 = Number To Boolean Array(number=w197) -> (Boolean array=w196:bool[])
        n588 = Number To Boolean Array(number=w194) -> (Boolean array=w195:bool[])
        n589 = Boolean Array To Number(Boolean array=w196) -> (number=w49:i32)
        n590 = Boolean Array To Number(Boolean array=w195) -> (number=w48:i32)
        n591 = case shown="True" "pow_fb" {
          tunnel: w69 -> [w295 w296]
          tunnel: [w295 w299] -> w68
          tunnel: w54 -> [_ w298]
          tunnel: "sum_z-pow_fb" -> [_ w297]
          frame False {
          }
          frame True {
            n592 = case shown="True" w297 {
              tunnel: [w300 w301] -> w299
              tunnel: w298 -> [w300 w303]
              tunnel: w296 -> [_ w302]
              frame False {
              }
              frame True {
                n593 = Add(x=w302, y=w303) -> (x+y=w301:i16)
              }
            }
          }
        }
        "z_fb_tot_i16" <- w68
        n594 = To Long Integer(number=w51) -> (32bit integer=w50:i32)
        n595 = Build Array(w191, w160, w161, w68, w49, w48) -> (w154:i32[])
        n596 = Build Array(w50, w49, w48) -> (w47:i32[])
        n597 = Build Array (concatenate)(w153, w154) -> (w152:i32[])
        n598 = xnode "FPGA I/O Node"("Connector0/AO0"=w160, "Connector0/AO1"=w161, "Connector0/AO3"=w68, "Connector0/AO6"=w68) -> ("Connector0/AI5"=w119:i16, "Connector0/AI6"=w120:i16)  [unwired: 6 in, 6 out]
        n599 = Build Array(w119, w119, w120) -> (w168:i16[])
      }
    }
  }
